vi "WS1050 36 DUT Reliability HD_Cycling_CP CVSweep_Ver1.0.vi"() -> ()   [LabVIEW 2012]
uses:
  WS_VCAP Driver 029/Source/WSVCAP Shell/Type Defs/WSVCAP SHL I2C DUT Mask Mode Enum.ctl
  <vilib>/Utility/file.llb/Read From Spreadsheet File (DBL).vi
panel:
  out "VISA out":refnum<visa-resource-name>="GPIB0::3::INSTR"
  out "error out 2":errorcluster={"status"=TRUE, "code"=-63192, "source"="niLvFpga_Open_PXI-7813R.vi"}
  in  "Reg1_Bit Cntrl":string[](array[string])=["01", "02", "04", "08", "10", "20", "40", "80", "03", "06", "0C", "D8", "33", "66", "CC", "07", "0E", "1C", "38", "70", "E0", "0F", "1E", "3C", "78", "F0", "1F", "3E", "7C", "F8", "3F", "7E", "FC", "7F", "FE", "FD", "FB", "F7", "EF", "DF", "BF", "7F", "FC", "F9", "F3", "E7", "CF", "9F", "3F", "F8", "F1", "E3", "C7", "8F", "1F", "F0", "E1", "C3", "87", "0F", "E0", "C1", "83", "07", "C0", "81", "03", "AA", "55", "00"]
  out "date string":string="5/19/2014"
  out "PS1 Out":refnum<visa-resource-name>
  out "Ke2000 Out":refnum<visa-resource-name>="GPIB0::9::INSTR"
  in  "VPI_Cmd":string[](array[string])=["00", "3B", "00"]
  in  "VPI Name":string[](array[string])=["All_Drivers OFF", "All Drivers ON", "All Drivers OFF2"]
  in  "Tab Control":T1(tab)
  in  "CP with DVA ON":i32(ring) items=["CP HDC 35V", "CP HDC 40.25V", "CP HDC 27.5V", "CP HDC 30.5V", "CP HDC 44V", "CP HDC 50V", "CP HDC 55V", "CP HDC 42.5V", "CP HDC 32V"]
  in  "No of Cmd":i64=2
  in  "Board#":string="BRD5"
  in  "Serial Number":string[][](table)=[["DUT", "SN"], ["DUT1", "1"], ["DUT2", "2"], ["DUT3", "3"], ["DUT4", "4"], ["DUT5", "5"], ["DUT6", "6"], ["DUT7", "7"], ["DUT8", "8"], ["DUT9", "9"], ["DUT10", "10"], ["DUT11", "11"], ["DUT12", "12"], ["DUT13", "13"], ["DUT14", "14"], ["DUT15", "15"], ["DUT16", "16"], ["DUT17", "17"], ["DUT18", "18"], ["DUT19", "19"], ["DUT20", "20"], ["DUT21", "21"], ["DUT22", "22"], ["DUT23", "23"], ["DUT24", "24"], ["DUT25", "25"], ["DUT26", "26"], ["DUT27", "27"], ["DUT28", "28"], ["DUT29", "29"], ["DUT30", "30"], ["DUT31", "31"], ["DUT32", "32"], ["DUT33", "33"], ["DUT34", "34"], ["DUT35", "35"], ["DUT36", "36"]]
  in  "SPI Clock Rate (Hz)":dbl=5000000.0 caption="Cycle Speed" format="%.1p Hz"
  in  "Wafer#":string="T7-EB"
  in  "File Name":string="CYC_WS1050_T7_EB_65C_40V_25DC_BRD5_150911_1"
  in  "TMN DC\\CAP Data Log File Path":path=path "C:/WS1050 36 DUT Data"
  in  "Test Program":string="WS1050 36 DUT HD_Cycling_CP CV Sweep Ver1.0"
  out "Current Date":string="8/28/2014"
  out "Current Time":string="0950"
  in  "Start Date":string="10/21/2014"
  in  "Start Time":string="1542"
  in  "Comment":string="CYC65C40V"
  in  "OK Button":bool
  in  "Calibration":bool
  in  "Verify CP":bool
  in  "CP Setting":i32(ring) items=["CP OFF", "CP ON", "CP 35V", "CP 40V", "DVA ON", "DVA OFF", "REG1 ON", "REG1 OFF", "REG2 ON", "REG2 OFF", "REG3 ON", "REG3 OFF"]
  in  "Set VDD":dbl=3.7 format="%.3g"
  in  "Command":string[](array[string])=["0702013B3B3B", "070201000000", "0702013B0000"]
  in  "Clock Rate (Hz)":dbl=1000000.0 caption="Meas Speed" format="%.1p Hz"
  out "AR  Measurent(Hz)":dbl
  in  "PS1 Source":refnum<visa-resource-name>="GPIB0::5::INSTR"
  in  "Ke2000":refnum<visa-resource-name>="GPIB0::9::INSTR"
  in  "CP to HD/Cycle":i32(ring)=1 items=["CP HDC 35V", "CP HDC 40.25V", "CP HDC 27.5V", "CP HDC 30.5V", "CP HDC 44V", "CP HDC 50V", "CP HDC 55V", "CP HDC 42.5V", "CP HDC 32V"]
  out "Simulate FPGA":bool
  out "Online":bool
  out "AR Cycling(Hz)":dbl=5000000.0
  in  "Ke2400":refnum<visa-resource-name>="GPIB0::3::INSTR"
  in  "Initialize AD7747":bool
  in  "DUT Mask Mode":T2=enum."All"
  in  "RFFE Slave Address":u8=7 caption="Slave Address" format="0x%02x"
  out "Activity Log":string="05/19/2014 -- 12:24:35.853::WSVCAP::APP::Application Started\n05/19/2014 -- 12:24:37.606::WSVCAP::WSVCAP SHL::WR I2C-REG:0x0A;MASK:0xFFFFFFFFFFFF;C1 DATA:22:22:22:22:22:22:22:22:22:22:22:22:22:22:22:22;C2 DATA:22:22:22:22:22:22:22:22:22:22:22:22:22:22:22:22;C3 DATA:22:22:22:22:22:22:22:22:22:22:22:22:22:22:22:22\r\n05/19/2014 -- 12:24:37.773::WSVCAP::WSVCAP SHL::WR I2C-ST:0,0,4,1\r\n05/19/2014 -- 12:24:37.903::WSVCAP::WSVCAP SHL::RD I2C-BYTES:4;ADD:0x00;MASK:0xFFFFFFFFFFFF\r\n05/19/2014 -- 12:24:38.045::WSVCAP::WSVCAP SHL::RD I2C:C1 DATA:2:2:2:2:2:2:2:2:2:2:2:2:2:2:2:2|A7:A9:AA:82:82:7F:82:81:82:81:83:82:81:82:82:81|46:36:BB:88:44:A3:E9:2B:32:20:ED:25:BB:3D:68:B|2C:6A:EB:A7:22:56:FE:CC:36:82:D7:B0:3B:48:F9:CC;C2 DATA:2:2:2:2:2:2:2:2:2:2:2:2:2:2:2:2|94:94:94:80:80:80:80:80:81:7E:7E:81:80:7E:80:80|47:33:15:82:62:B:E8:1C:D7:C3:7D:41:7C:B7:4C:2A|C4:B4:AE:8:1E:D1:4E:37:11:C0:6F:63:42:9D:63:B5;C3 DATA:2:2:2:2:2:2:2:2:2:2:2:2:2:2:2:2|95:95:95:81:81:7E:81:80:84:7D:80:83:81:7E:7F:80|AB:C4:14:B5:7B:52:DF:C9:79:5D:5F:30:99:31:1E:F4|6E:5C:F7:A8:C3:EB:7B:EF:33:92:89:77:4D:67:75:DD;STATUS:0:0:4:0\r\n05/19/2014 -- 12:24:38.046::WSVCAP::WSVCAP SHL::WR I2C-REG:0x0A;MASK:0xFFFFFFFFFFFF;C1 DATA:22:22:22:22:22:22:22:22:22:22:22:22:22:22:22:22;C2 DATA:22:22:22:22:22:22:22:22:22:22:22:22:22:22:22:22;C3 DATA:22:22:22:22:22:22:22:22:22:22:22:22:22:22:22:22\r\n05/19/2014 -- 12:24:38.089::WSVCAP::WSVCAP SHL::WR I2C-ST:0,0,4,1\r\n05/19/2014 -- 12:24:38.219::WSVCAP::WSVCAP SHL::RD I2C-BYTES:4;ADD:0x00;MASK:0xFFFFFFFFFFFF\r\n05/19/2014 -- 12:24:38.362::WSVCAP::WSVCAP SHL::RD I2C:C1 DATA:2:2:2:2:2:2:2:2:2:2:2:2:2:2:2:2|A7:AB:AA:82:82:82:83:83:82:82:82:82:7F:82:82:81|4B:32:96:83:3E:61:43:17:25:62:AB:4D:A2:40:2E:5|3C:76:2B:B4:EE:E4:A9:1A:AA:A:26:C7:21:2E:87:5B;C2 DATA:2:2:2:2:2:2:2:2:2:2:2:2:2:2:2:2|94:94:94:80:80:80:80:80:80:7F:80:81:80:80:7F:80|4A:32:19:7D:19:6C:79:46:61:7F:4B:B8:A5:30:F3:14|B4:70:A:8C:9C:DC:43:FA:1E:A:C6:21:A:A9:13:F3;C3 DATA:2:2:2:2:2:2:2:2:2:2:2:2:2:2:2:2|95:97:94:81:80:81:82:81:80:7E:81:84:7F:81:80:80|B2:32:D0:A7:9E:4C:AB:D4:EE:D9:F0:82:B7:91:7:FF|C1:91:B6:3D:D8:E:1B:4F:9F:6A:F1:6C:E7:3F:7:BA;STATUS:0:0:4:0\r\n05/19/2014 -- 12:24:38.364::WSVCAP::WSVCAP SHL::WR I2C-REG:0x0A;MASK:0xFFFFFFFFFFFF;C1 DATA:22:22:22:22:22:22:22:22:22:22:22:22:22:22:22:22;C2 DATA:22:22:22:22:22:22:22:22:22:22:22:22:22:22:22:22;C3 DATA:22:22:22:22:22:22:22:22:22:22:22:22:22:22:22:22\r\n05/19/2014 -- 12:24:38.406::WSVCAP::WSVCAP SHL::WR I2C-ST:0,0,4,1\r\n05/19/2014 -- 12:24:38.536::WSVCAP::WSVCAP SHL::RD I2C-BYTES:4;ADD:0x00;MASK:0xFFFFFFFFFFFF\r\n05/19/2014 -- 12:24:38.678::WSVCAP::WSVCAP SHL::RD I2C:C1 DATA:2:2:2:2:2:2:2:2:2:2:2:2:2:2:2:2|A7:A9:AB:82:82:81:82:82:82:82:82:82:82:82:82:81|46:71:4C:87:43:3D:7F:FC:25:4F:8E:54:97:3E:60:8C|AA:F4:1F:B5:CE:43:1F:36:9:87:9C:78:86:5:B6:8E;C2 DATA:2:2:2:2:2:2:2:2:2:2:2:2:2:2:2:2|94:94:94:80:7F:7F:80:80:80:80:80:81:80:80:80:80|49:36:18:7D:6E:C5:E4:3C:81:2E:41:D3:75:71:E3:72|E8:D3:E6:D1:E0:48:AE:D4:54:D:E8:8E:B4:41:68:4;C3 DATA:2:2:2:2:2:2:2:2:2:2:2:2:2:2:2:2|95:95:95:81:7F:7F:81:81:81:81:81:84:81:81:82:81|B3:F5:90:AB:82:69:7B:93:D0:77:E8:D5:E8:8C:84:E8|B9:AC:EE:2B:B6:71:8F:4A:74:31:56:BB:8A:B7:A0:C8;STATUS:0:0:4:0\r\n05/19/2014 -- 12:24:38.681::WSVCAP::WSVCAP SHL::WR I2C-REG:0x0A;MASK:0xFFFFFFFFFFFF;C1 DATA:22:22:22:22:22:22:22:22:22:22:22:22:22:22:22:22;C2 DATA:22:22:22:22:22:22:22:22:22:22:22:22:22:22:22:22;C3 DATA:22:22:22:22:22:22:22:22:22:22:22:22:22:22:22:22\r\n05/19/2014 -- 12:24:38.723::WSVCAP::WSVCAP SHL::WR I2C-ST:0,0,4,1\r\n05/19/2014 -- 12:24:38.854::WSVCAP::WSVCAP SHL::RD I2C-BYTES:4;ADD:0x00;MASK:0xFFFFFFFFFFFF\r\n05/19/2014 -- 12:24:38.996::WSVCAP::WSVCAP SHL::RD I2C:C1 DATA:2:2:2:2:2:2:2:2:2:2:2:2:2:2:2:2|A7:A9:AA:82:82:7F:83:81:82:81:84:82:7F:82:7F:82|43:FB:E:7F:3C:AD:35:35:26:A2:6C:21:4B:3D:8:6|63:9A:E1:F3:95:32:91:42:90:3C:78:1F:5C:D7:5F:D8;C2 DATA:2:2:2:2:2:2:2:2:2:2:2:2:2:2:2:2|94:94:94:80:80:80:80:80:81:80:7E:81:80:7E:7F:80|48:36:18:7F:5E:3D:69:83:DE:AE:A1:9E:31:AE:BB:96|15:A0:44:17:13:FD:CC:C8:6D:B2:EF:A7:C:C7:3B:F;C3 DATA:2:2:2:2:2:2:2:2:2:2:2:2:2:2:2:2|95:96:94:81:81:7E:82:80:84:80:80:84:7F:7E:7D:82|AD:3B:6D:A9:7C:57:9D:F5:7A:96:23:5C:36:2D:ED:5A|CD:46:DB:3B:C7:BD:70:60:33:B8:B:F7:63:A:51:4D;STATUS:0:0:4:0\r\n05/19/2014 -- 12:24:38.998::WSVCAP::WSVCAP SHL::WR I2C-REG:0x0A;MASK:0xFFFFFFFFFFFF;C1 DATA:22:22:22:22:22:22:22:22:22:22:22:22:22:22:22:22;C2 DATA:22:22:22:22:22:22:22:22:22:22:22:22:22:22:22:22;C3 DATA:22:22:22:22:22:22:22:22:22:22:22:22:22:22:22:22\r\n05/19/2014 -- 12:24:39.040::WSVCAP::WSVCAP SHL::WR I2C-ST:0,0,4,1\r\n05/19/2014 -- 12:24:39.170::WSVCAP::WSVCAP SHL::RD I2C-BYTES:4;ADD:0x00;MASK:0xFFFFFFFFFFFF\r\n05/19/2014 -- 12:24:39.311::WSVCAP::WSVCAP SHL::RD I2C:C1 DATA:2:2:2:2:2:2:2:2:2:2:2:2:2:2:2:2|A7:AA:AB:82:82:81:82:81:82:81:82:82:82:82:7F:82|44:F1:90:87:45:44:C8:2C:2C:F1:FC:1B:94:3B:3C:75|4A:49:95:19:99:73:64:3:23:24:F3:A2:5E:7F:C4:B6;C2 DATA:2:2:2:2:2:2:2:2:2:2:2:2:2:2:2:2|94:94:94:80:80:80:80:7F:80:80:7E:80:80:7E:7F:80|4C:36:17:7D:A8:9F:DE:C7:53:6D:8A:F4:41:A5:C6:E0|90:2E:24:C:D9:22:E4:76:3B:40:1D:53:33:B1:3E:4D;C3 DATA:2:2:2:2:2:2:2:2:2:2:2:2:2:2:2:2|95:97:95:81:81:7F:81:80:80:81:7F:82:81:7E:7D:82|AE:2B:A7:AB:CC:CD:A4:38:FD:17:80:F2:92:2D:45:C4|76:E5:D:B9:AD:B5:BA:8D:28:32:9E:42:B7:20:4A:D9;STATUS:0:0:4:0\r\n05/19/2014 -- 12:24:39.313::WSVCAP::WSVCAP SHL::WR I2C-REG:0x0A;MASK:0xFFFFFFFFFFFF;C1 DATA:22:22:22:22:22:22:22:22:22:22:22:22:22:22:22:22;C2 DATA:22:22:22:22:22:22:22:22:22:22:22:22:22:22:22:22;C3 DATA:22:22:22:22:22:22:22:22:22:22:22:22:22:22:22:22\r\n05/19/2014 -- 12:24:39.355::WSVCAP::WSVCAP SHL::WR I2C-ST:0,0,4,1\r\n05/19/2014 -- 12:24:39.486::WSVCAP::WSVCAP SHL::RD I2C-BYTES:4;ADD:0x00;MASK:0xFFFFFFFFFFFF\r\n05/19/2014 -- 12:24:39.628::WSVCAP::WSVCAP SHL::RD I2C:C1 DATA:2:2:2:2:2:2:2:2:2:2:2:2:2:2:2:2|A7:A9:AA:82:82:82:83:82:82:82:82:82:7F:82:7F:82|47:18:E4:87:3E:E7:6:65:25:92:37:38:A8:3E:89:85|7C:A7:7:2B:A3:7A:EC:EF:89:ED:F4:D3:D8:BC:3A:F5;C2 DATA:2:2:2:2:2:2:2:2:2:2:2:2:2:2:2:2|94:94:94:80:7F:80:80:7F:81:80:7E:80:80:80:81:80|49:37:17:80:76:25:6A:F8:DF:55:97:4D:B8:5B:2B:B1|13:E3:9A:3E:1A:2D:4F:B6:DB:E9:61:FA:8B:D6:9:CC;C3 DATA:2:2:2:2:2:2:2:2:2:2:2:2:2:2:2:2|95:95:95:81:7F:80:82:81:84:80:7F:81:80:81:7F:82|AF:93:3B:AF:5B:11:82:E4:7E:C3:2D:72:9:96:D9:A|DB:96:F2:10:5F:64:9A:C6:98:12:27:7D:10:D3:20:D9;STATUS:0:0:4:0\r\n05/19/2014 -- 12:24:40.132::WSVCAP::WSVCAP SHL::CLOSE\r\n"
  in  "C1 Cap DAC":u8=128 caption="B Data In" format="0x%02x"
  in  "C2 Cap DAC":u8=128 caption="B Data In" format="0x%02x"
  in  "C3 Cap DAC":u8=128 caption="B Data In" format="0x%02x"
  out "IDD Brd(uA)":string
  in  "Repeat Meas(s)":u32=900
  in  "Real No. From\nLookup Table":bool
  in  "Control Panel":T3={"Verify Socket"=FALSE, "HD/CYC"=FALSE, "E-CAL"=FALSE, "DVA"=FALSE, "VPI"=TRUE, "VSA"=TRUE, "HS"=FALSE}
  out "Verify Socket":bool
  out "HD/CYC":bool
  out "E-CAL":bool
  out "DVA":bool
  out "VPI":bool
  out "VSA":bool
  out "HS":bool
  in  "Lot#":string="WS1050"
  out "AD7747 Values":string[][](table)
  in  "Freq(Hz)":string="12K"
  in  "Reset P/S":bool
  in  "Test Sequences":i32(ring) items=["C1_C2_C3", "C2_C1_C3", "C3_C2_C1"]
  in  "WS1050/51":bool=TRUE
  in  "% Duty Cycle":string="25"
  in  "Cmd To HD":string="0702013B3B3B"
  in  "Post CMd Delay":dbl[](array[numeric])=[1.7e-05, 5.4e-05, 1.8e-05] min=0.0 max=0.5 format="%#.0p s"
  in  "Cmin/Act":bool=TRUE
  in  "CP to Meas":i32(ring)=1 items=["CP HDC 35V", "CP HDC 40.25V", "CP HDC 27.5V", "CP HDC 30.5V", "CP HDC 44V", "CP HDC 50V", "CP HDC 55V", "CP HDC 42.5V", "CP HDC 32V"]
  in  "CP VPI":i32(ring) items=["CP HDC 35V", "CP HDC 40.25V", "CP HDC 27.5V", "CP HDC 30.5V", "CP HDC 44V", "CP HDC 50V", "CP HDC 55V", "CP HDC 42.5V", "CP HDC 32V"]
  out "CAP_C1":string[][](table)
  out "NOM IDD OFF(uA)":string
  out "CAP_C2":string[][](table)
  out "CAP_C3":string[][](table)
  out "Total Time":u64
  in  "Set HD/Cycle \nto Complete":u64=5000000000
  out "No of HD/Cycle\nCompleted":u64
  out "Cycle Count":u64 min=1 max=4 step=1
  out "Loop \ncompleted":i32=1
  out "Previous Time":string="12:20:26 PM"
  out "STATUS":string="Idle...."
  out "Total Delta C2(pF)":string[](array[string])
  out "Total Delta C1(pF)":string[](array[string])
  out "Total Delta C3(pF)":string[](array[string])
  out "RB Reg for HD":string[](array[string])
  out "RB Reg for HD/Cycle":string[](array[string])
  out "VPI C2":string[][](table)
  out "VPI C3":string[][](table)
  out "NOM IDD ON (uA)":string
  out "IDD_HD/CYC (uA)":string="164.601255E+0"
  in  "stop During HD/Cycles":bool
  in  "stop":bool
  out "IDD Stdby(uA)":string="2.606990E+0"
  out "VPI C1":string[][](table)
  out "VSA_V1":string[][](table)
  out "VSA_V2":string[][](table)
  out "VSA_V3":string[][](table)
  in  "VSA Voltage(V)":dbl[](array[numeric])=[-10.0, 0.0, 10.0]
  in  "DC_Temp":i32=65
  in  "HD/CYC Temp":i32=65
  in  "Time All ON (s)":u32=120
  in  "Time All OFF (s)":u32=120
  in  "HD_DC (Min)":u64=259200
  out "LPs Count":i32
  in  "X Repeat":i32=100
  out "No LPs to RP":i32
  out "Run Loops":i32=1
  out "TTCompleted":u64=2000
  in  "TTF Completed":u64=5000000000
  out "% Delta C_T0":string[][](array[string])
  out "% Delta C":string[][](array[string])
  out "EFuse RB T0":string[](array[string])
  out "Current EFuse Read back":string[](array[string])
  out "EFuse Readback Status":bool[](array[boolean])
  in  "DeltaC Target Setting(pF)":dbl=7.375
  out "error out":errorcluster
  in  "error in (no error)":errorcluster
  in  "HD RP":dbl=60.0
  in  "Cycle RP":dbl=10000.0
  out "Min Plot_1":dbl[][](graph) caption="(Y) Multi Plot 2"
  out "Min Plot_2":dbl[][](graph) caption="(Y) Multi Plot 2"
  out "Min Plot_3":dbl[][](graph) caption="(Y) Multi Plot 2"
  in  "Debug":bool
  in  "No of Rows\nFrom Spread Sheet":i32
  in  "Plot Delta Cmin":bool=TRUE
  in  "Plot":T4(ring)
  in  "Bank C1":i32(ring) items=["C1", "C2", "C3", "D_C1", "D_C2", "D_C3"]
  in  "Bank C2":i32(ring)=1 items=["C1", "C2", "C3", "D_C1", "D_C2", "D_C3"]
  in  "Bank C3":i32(ring)=2 items=["C1", "C2", "C3", "D_C1", "D_C2", "D_C3"]
  in  "Manual Setting\nFor RP CP CV":i64[](array[numeric])=[0, 100000, 5000000]
  in  "CP CV \nSweep":bool=TRUE
  out "CP CV Sweep C1":dbl[][](graph) caption="(Y) Multi Plot 2"
  out "CP CV Sweep C2":dbl[][](graph) caption="(Y) Multi Plot 2"
  out "CP CV Sweep C3":dbl[][](graph) caption="(Y) Multi Plot 2"
  out "LP CP Voltage":string
  in  "Auto\nMan":bool
  in  "Start":i64
  in  "Stop":i64
  in  "Step":i64
  out "RP for CP CV":i64[](array[numeric])
  out "CP to Run":dbl[](array[numeric])
  # "Company:  WiSpry Inc\n20 Fairbanks Ste 198 Irvine CA 92618\n\nAuthor:  Andy V Tran\nCreated:  09/14/2015\nLabVIEW 2012 Pro\nTest Program:  WS1050 36 DUT Reliability HD_Cycling CP CV Sweep ver1.0\nFPGA: WS_VCAP Driver 029"
  # "Note for HD Duty Cycle:\n1.  Set time to start HD_DC (Min), default is 259200 (6 months) \n2.  Set Time for Duty Cycle ON/OFF, default setting is 2 minutes\n3.  No of Loops to RP = 3600s/(Time ALL ON(s) + Time ALL + OFF(s))\n4.  Set X Repeat = no of runs, default is 100 runs\n5.  Set TTF Completed to stop the test.\n\nVer 1.0:\n1.  Original version, set CP voltage measure all drivers"
  # "Minutes"
  # "X1000"
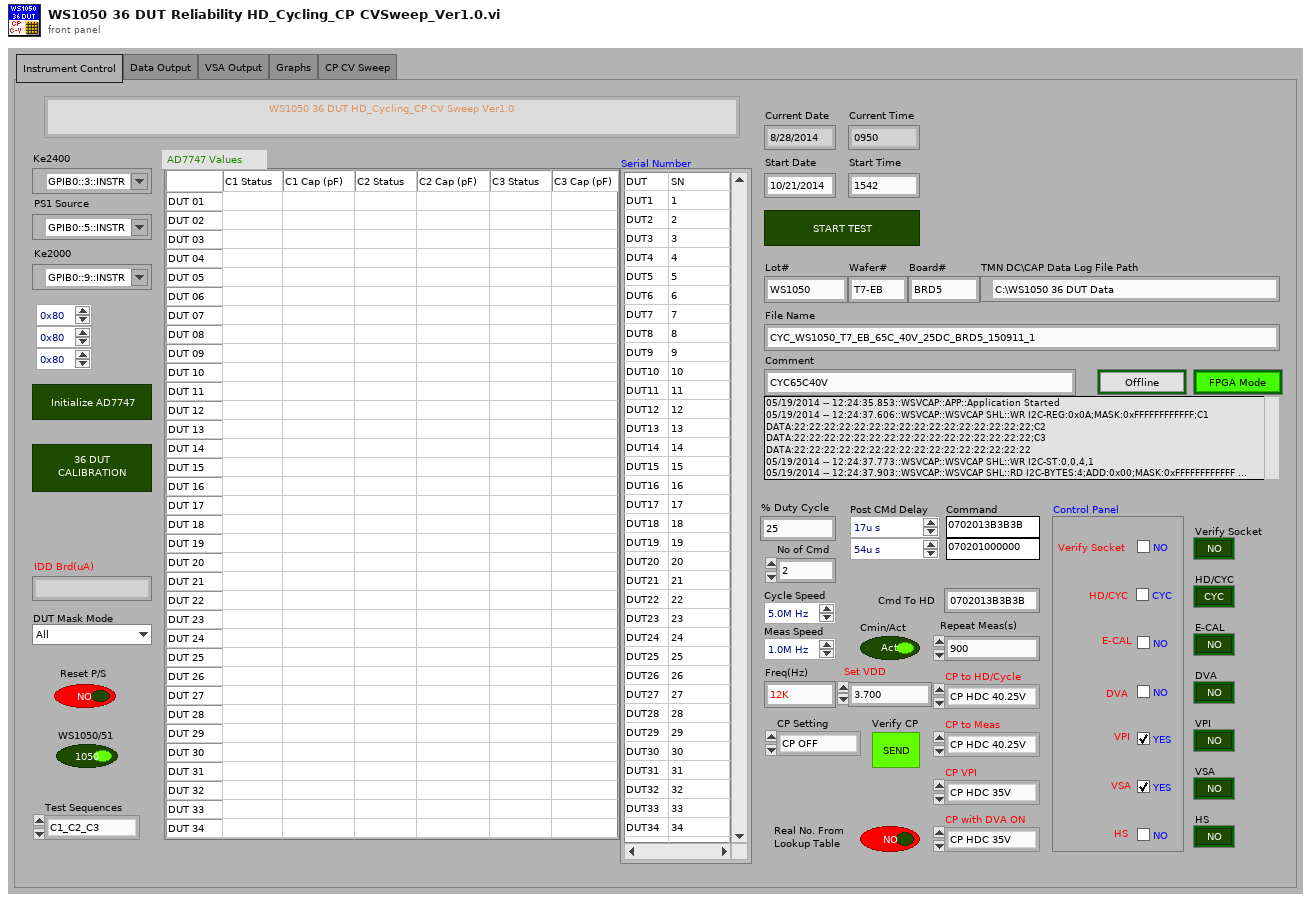
[diagram p1: front panel]
types:
  T1 = enum32{"Instrument Control", "Data Output", "VSA Output", "Graphs", "CP CV Sweep"}
  T2 = typedef "WSVCAP SHL I2C DUT Mask Mode Enum.ctl" = enum16{"Custom", "C1", "C2", "C3", "All"}
  T3 = cluster{"Verify Socket":bool, "HD/CYC":bool, "E-CAL":bool, "DVA":bool, "VPI":bool, "VSA":bool, "HS":bool}
  T4 = enum16{"ALL DUTs", "DUT 01", "DUT 02", "DUT 03", "DUT 04", "DUT 05", "DUT 06", "DUT 07", "DUT 08", "DUT 09", "DUT 10", "DUT 11", "DUT 12", "DUT 13", "DUT 14", "DUT 15", "DUT 16", "DUT 17", "DUT 18", "DUT 19", "DUT 20", "DUT 21", "DUT 22", "DUT 23", "DUT 24", "DUT 25", "DUT 26", "DUT 27", "DUT 28", "DUT 29", "DUT 30", "DUT 31", "DUT 32", "DUT 33", "DUT 34", "DUT 35", "DUT 36"}
  T5 = typedef "WSVCAP SHL Core System Cluster.ctl" = cluster{"Settings":T6, "FPGA Resource":tag, "Online":bool, "I2C Wait Ticks":u32, "SPI Wait Ticks":u32, "RFFE Wait Ticks":u32}
  T6 = typedef "WSVCAP SHL I2C Settings Cluster.ctl" = cluster{"FPGA Resource Name":string, "I2C Slave Address":u8, "I2C Clock Rate (Hz)":dbl, "SPI Clock Rate (Hz)":dbl, "RFFE Slave Address":u8, "RFFE Clock Rate (Hz)":dbl, "Simulate FPGA":bool, "C1 Cap DAC Default":u8, "C2 Cap DAC Default":u8, "C3 Cap DAC Default":u8}
  T7 = enum16{"Idle...", "Voltage 1", "Voltage 2", "Voltage 3"}[]
  T8 = cluster{"Test Program ":string, "Comment":string, "Data Out":string, "Data Out":string, "Data Out":string, string, "Data Out":string, "Data Out":string, "Data Out":string, "Freq(Hz)":string, "Board#":string}
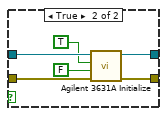
[diagram p2: hidden frame]
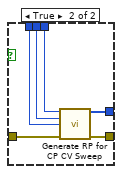
[diagram p8: hidden frame]
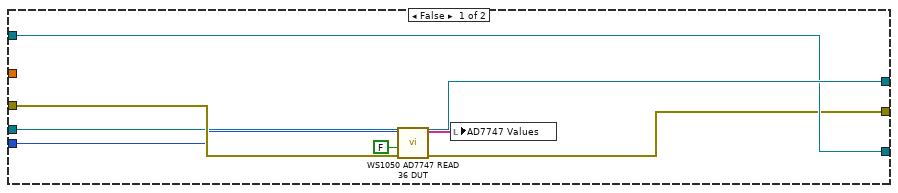
[diagram p11: hidden frame]
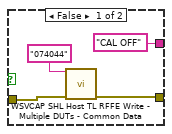
[diagram p12: hidden frame]
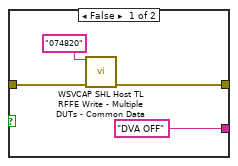
[diagram p13: hidden frame]
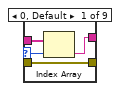
[diagram p14: hidden frame]
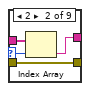
[diagram p15: hidden frame]
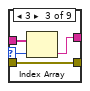
[diagram p16: hidden frame]
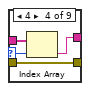
[diagram p17: hidden frame]
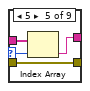
[diagram p18: hidden frame]
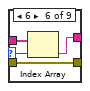
[diagram p19: hidden frame]
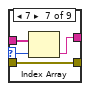
[diagram p20: hidden frame]
diagram:
  w26 = TRUE
  w30 = u16 0 items=["Off", "Moving Filter", "Repeating Filter"] ("Digital Filter (0: Off)")
  w31 = u16 7 items=["3.5 Digits"=4, "4.5 Digits"=5, "5.5 Digits"=6, "6.5 Digits"=7] ("Resolution (7: 6.5 digits)")
  n1 = case shown="True" w26 {
    tunnel: "error in (no error)" -> [w38 w39]
    tunnel: [w38 w46] -> w15
    frame False {
    }
    frame True {
      n2 = call "WSVCAP SHL Host TL Initialize.vi"("error in"=w39) -> ("error out"=w40:errorcluster)  [unwired: 13 in, 1 out]
      n3 = control-ref of="Activity Log"() -> (w42:refnum<vi>)
      n4 = call "ACT LG Activity Log Core.vi"("Display Ref"=w42, "Source"="WSVCAP", "Error In (no error)"=w40) -> ("Error Out"=w41:errorcluster)  [unwired: 11 in, 1 out]
      n5 = call "WSVCAP SHL Host TL Status Manager.vi"("error in"=w41) -> ("System Out"=w47:T5, "error out"=w46:errorcluster)  [unwired: 13 in]
      n6 = Unbundle By Name(w47) -> ("Online"=→"Online":bool, "Settings.Simulate FPGA"=→"Simulate FPGA":bool)
    }
  }
  n7 = case shown="True" TRUE {
    tunnel: [_ w50] -> w37
    tunnel: [_ w48] -> w1
    frame False {
    }
    frame True {
      n8 = flat-sequence {
        tunnel: [w51] -> w49
        tunnel: [w55] -> w50
        tunnel: w49 -> [w55]
        tunnel: [w53] -> w48
        frame #0 {
          n9 = call-poly <vilib>:"Read From Spreadsheet File.vi"("number of rows (all:-1)"=-1) -> ("all rows"=w51:dbl[][])  [unwired: 6 in, 4 out]
        }
        frame #1 {
          n10 = call-poly <vilib>:"Read From Spreadsheet File.vi"("number of rows (all:-1)"=-1) -> ("all rows"=w53:dbl[][])  [unwired: 6 in, 4 out]
        }
      }
    }
  }
  n11 = case shown="True" TRUE {
    tunnel: w15 -> [w56 w61]
    tunnel: [w57 w60] -> w23
    tunnel: [w56 w59] -> w19
    tunnel: "Ke2400" -> [w57 w58]
    frame False {
    }
    frame True {
      n12 = VISA Write(VISA resource name=w58, write buffer="SOUR:FUNC VOLT;VOLT:MODE FIX;RANG 100;LEV 0.0;:SENS:FUNC \"CURR\";CURR:PROT 60E-3;RANG 100E-3;:OUTP ON", error in (no error)=w61) -> (VISA resource name out=w60:refnum<visa-resource-name>, error out=w59:errorcluster)  [unwired: 1 out]
    }
  }
  n13 = case shown="False" "Reset P/S" {
    tunnel: "PS1 Source" -> [w63 w70]
    tunnel: [w63 w68] -> w35
    tunnel: w15 -> [w64 w66]
    tunnel: [w64 w65] -> w14
    frame False {
    }
    frame True {
      n14 = call "Agilent 3631A Initialize.vi"("error in (no error)"=w66, "Default"=FALSE ("Reset? (T: Yes)"), "Reset"=TRUE ("ID Query? (T: Yes)"), "VISA resource name"=w70) -> ("error out"=w65:errorcluster, "VISA resource name out"=w68:refnum<visa-resource-name>)  [unwired: 6 in]
    }
  }
  n15 = call "Ke2000 Initialize.vi"("error in (no error)"=w15, "VISA resource name"="Ke2000") -> ("error out"=w32:errorcluster, "VISA resource name out"=w33:refnum<visa-resource-name>)  [unwired: 8 in]
  n16 = call "Ke2000 Configure DC Current.vi"("Resolution (7: 6.5 digits)"=w31, "Digital Filter (0: Off)"=w30, "Auto Range? (T: Auto)"=FALSE, "error in"=w32, "Custom Range (0 A)"=1.0, "VISA resource name"=w33) -> ("error out"=w16:errorcluster, "VISA resource name out"=w28:refnum<visa-resource-name>)  [unwired: 4 in]
  n17 = Merge Errors(w19, w16, w14) -> (w24:errorcluster)
  n18 = while {
    tunnel: w24 -> [w79]
    tunnel: [w75] -> w5
    tunnel: w37 -> [w102]
    tunnel: w35 -> [w90]
    tunnel: w28 -> [w91]
    tunnel: [w100] -> w11
    tunnel: [w99] -> w6
    tunnel: w23 -> [w97]
    tunnel: [w96] -> w21
    tunnel: [FALSE ("stop")] -> w17
    tunnel: w1 -> [w72]
    i -> [w98]
    stop <- w103 stop-if-true
    n19 = case shown="0" w98 {
      tunnel: w79 -> [w113 w115]
      tunnel: [w112 w115] -> w93
      tunnel: "RFFE Slave Address" -> [w110 _]
      frame 0 {
        w106 = dbl[][] []
        w105 = "" ("uA")
        w107 = string[][] []
        w108 = string[] [] ("EFuse Read back")
        w114 = u64 0 ("No of HD/Cycle\nCompleted")
        n20 = local write "RB Reg for HD/Cycle"(w108) -> ()
        n21 = local write "Current EFuse Read back"(w108) -> ()
        n22 = local write "EFuse RB T0"(w108) -> ()
        n23 = local write "Total Delta C1(pF)"(w108) -> ()
        n24 = local write "Total Delta C2(pF)"(w108) -> ()
        n25 = local write "Total Delta C3(pF)"(w108) -> ()
        n26 = local write "No of HD/Cycle\nCompleted"(w114) -> ()
        n27 = local write "Cycle Count"(w114) -> ()
        n28 = local write "CAP_C2"(w107) -> ()
        n29 = local write "CAP_C1"(w107) -> ()
        n30 = local write "VPI C2"(w107) -> ()
        n31 = local write "VSA_V3"(w107) -> ()
        n32 = local write "VSA_V1"(w107) -> ()
        n33 = local write "NOM IDD OFF(uA)"(w105) -> ()
        n34 = local write "NOM IDD ON (uA)"(w105) -> ()
        n35 = local write "IDD Brd(uA)"(w105) -> ()
        n36 = local write "CAP_C3"(w107) -> ()
        n37 = local write "VSA_V2"(w107) -> ()
        n38 = local write "VPI C1"(w107) -> ()
        n39 = local write "VPI C3"(w107) -> ()
        n40 = local write "% Delta C"(w107) -> ()
        n41 = local write "% Delta C_T0"(w107) -> ()
        n42 = call "WSVCAP SHL Host TL RFFE Configure.vi"("RFFE Slave Address"=w110, "Clock Rate (Hz)"="Clock Rate (Hz)", "error in"=w113) -> ("Actual Rate (Hz)"=→"AR  Measurent(Hz)":dbl, "error out"=w112:errorcluster)  [unwired: 11 in]
        n43 = local write "Min Plot_3"(w106) -> ()
        n44 = local write "Min Plot_1"(w106) -> ()
        n45 = local write "Min Plot_2"(w106) -> ()
      }
      frame 1, Default {
      }
    }
    n46 = while {
      tunnel: ["stop"] -> w95
      tunnel: w93 -> [w152]
      tunnel: [w121] -> w87
      tunnel: w90 -> [w151]
      tunnel: w91 -> [w146]
      tunnel: [w147] -> w89
      tunnel: [w145] -> w88
      tunnel: [w143] -> w86
      tunnel: [w142] -> w85
      tunnel: [w141] -> w84
      tunnel: [w140] -> w83
      tunnel: [w139] -> w82
      tunnel: [w138] -> w81
      tunnel: [w137] -> w80
      tunnel: ["Command"] -> w78
      tunnel: ["Post CMd Delay"] -> w77
      tunnel: "Set VDD" -> [w127]
      tunnel: [w116] -> w71
      stop <- w159 stop-if-true
      # "Set Date & Time to Start Test"
      n47 = case shown="True" "Initialize AD7747" {
        tunnel: w152 -> [w176 w182]
        tunnel: [w176 w178] -> w136
        tunnel: w151 -> [w175 w180]
        tunnel: [w175 w179] -> w150
        tunnel: w127 -> [_ w177]
        frame False {
        }
        frame True {
          w183 = T7 [enum."Voltage 2", enum."Voltage 3", enum."Voltage 1"] items=["Idle...", "Voltage 1", "Voltage 2", "Voltage 3"]
          n48 = for {
            tunnel: w180 -> [w193]
            tunnel: w183 -> [w191] mode=indexing
            tunnel: [w190] -> w179
            shift-right: [w187] -> w181
            shift-left: w182 -> [w194]
            tunnel: w177 -> [w184]
            n49 = call "E3631A_Voltage Controller updated.vi"("VISA resource name"=w193, "I_VDD(A)"=0.5, "Channel Controller"=w191, "Voltage 1"=w184, "Voltage 2"=3.3, "error in (no error)"=w194, "I_3.3V (A)"=0.5) -> ("VISA resource name out"=w190:refnum<visa-resource-name>, "error out"=w186:errorcluster)  [unwired: 7 in]
            n50 = call "Delay.vi"("milliseconds to wait"=u32 100, "error in (no error)"=w186) -> ("error out"=w187:errorcluster)  [unwired: 9 in]
          }
          n51 = call "WS1050_AD7747_Init 36DUT.vi"("error in"=w181) -> ("error out"=w178:errorcluster)  [unwired: 10 in]
        }
      }
      n52 = call "Time_stamp.vi"() -> ("date/time string"=w164:string, "date string"=w166:string)  [unwired: 2 in]
      "Current Date" <- w166
      "Current Time" <- w164
      n53 = Equal?(x=w166, y="Start Date") -> (x = y?=w162:bool)
      n54 = Equal?(x=w164, y="Start Time") -> (x = y?=w161:bool)
      n55 = And(x=w162, y=w161) -> (x .and. y?=w158:bool)
      n56 = Compound Arithmetic op=OR(w158, "OK Button", "stop") -> (w159:bool)
      n57 = case shown="True" "Calibration" {
        tunnel: w136 -> [w225 w243]
        tunnel: [w219 w240] -> w134
        tunnel: w150 -> [w224 w239]
        tunnel: "DUT Mask Mode" -> [w223 w235]
        tunnel: [w224 w234] -> w148
        tunnel: w146 -> [w222 w233]
        tunnel: [w222 w230] -> w145
        tunnel: w127 -> [_ w229]
        tunnel: "C1 Cap DAC" -> [_ w228]
        tunnel: "C2 Cap DAC" -> [_ w227]
        tunnel: "C3 Cap DAC" -> [_ w226]
        frame False {
          n58 = call "WS1050 AD7747 READ 36 DUT.vi"("error in"=w225, "Log (T)"=FALSE, "DUT Mask Mode (All)"=w223) -> ("error out"=w219:errorcluster, "AD7747 Values"=w220:string[][])  [unwired: 7 in]
          n59 = local write "AD7747 Values"(w220) -> ()
        }
        frame True {
          n60 = flat-sequence {
            tunnel: w243 -> [w253]
            tunnel: [w248] -> w242
            tunnel: w239 -> [w252]
            tunnel: [w251] -> w238
            tunnel: w235 -> [w250]
            tunnel: [w250] -> w236
            tunnel: w233 -> [w246]
            tunnel: [w245] -> w232
            tunnel: w229 -> [w244]
            tunnel: w242 -> [w279]
            tunnel: [w278] -> w241
            tunnel: w238 -> [w277]
            tunnel: [w277] -> w237
            tunnel: w236 -> [w276]
            tunnel: w228 -> [w272]
            tunnel: w227 -> [w271]
            tunnel: w226 -> [w270]
            tunnel: w232 -> [w269]
            tunnel: [w269] -> w231
            tunnel: w241 -> [w282]
            tunnel: [w285] -> w240
            tunnel: w237 -> [w284]
            tunnel: [w281] -> w234
            tunnel: w231 -> [w280]
            tunnel: [w280] -> w230
            frame #0 {
              w254 = T7 [enum."Voltage 2", enum."Voltage 3", enum."Voltage 1"] items=["Idle...", "Voltage 1", "Voltage 2", "Voltage 3"]
              n61 = for {
                tunnel: w252 -> [w265]
                tunnel: w254 -> [w263] mode=indexing
                tunnel: [w262] -> w251
                shift-right: [w260] -> w247
                shift-left: w253 -> [w266]
                tunnel: w244 -> [w256]
                n62 = call "E3631A_Voltage Controller updated.vi"("VISA resource name"=w265, "I_VDD(A)"=0.5, "Channel Controller"=w263, "Voltage 1"=w256, "Voltage 2"=3.3, "error in (no error)"=w266, "I_3.3V (A)"=0.5) -> ("VISA resource name out"=w262:refnum<visa-resource-name>, "error out"=w259:errorcluster)  [unwired: 7 in]
                n63 = call "Delay.vi"("milliseconds to wait"=u32 100, "error in (no error)"=w259) -> ("error out"=w260:errorcluster)  [unwired: 9 in]
              }
              n64 = call "Ke2000 Single Reading.vi"("error in (no error)"=w247, "VISA resource name"=w246) -> ("error out"=w248:errorcluster, "VISA resource name out"=w245:refnum<visa-resource-name>, "uA"=→"IDD Brd(uA)":string)  [unwired: 5 in, 2 out]
              n65 = One Button Dialog(message="Please verify all sockets should be empty...") -> ()  [unwired: 1 in, 1 out]
            }
            frame #1 {
              n66 = call "WS1050 CAPDAC Setting.vi"("DUT Mask Mode (All)"=w276, "error in"=w279, "C3 Cap DAC"=w270, "C2 Cap DAC"=w271, "C1 Cap DAC"=w272) -> ("error out"=w274:errorcluster)  [unwired: 6 in]
              n67 = call "WS1050 OFFSET CAL updated.vi"("error in"=w274, "OFFSET CAL"=TRUE ("Read?")) -> ("error out"=w273:errorcluster)  [unwired: 9 in]
              n68 = call "WS1050 AD7747 READ 36 DUT.vi"("error in"=w273, "Log (T)"=FALSE, "DUT Mask Mode (All)"=w276) -> ("error out"=w278:errorcluster, "AD7747 Values"=→"AD7747 Values":string[][])  [unwired: 7 in]
            }
            frame #2 {
              w283 = T7 [enum."Voltage 2", enum."Voltage 3", enum."Voltage 1"] items=["Idle...", "Voltage 1", "Voltage 2", "Voltage 3"]
              n69 = for {
                tunnel: w284 -> [w297]
                tunnel: w283 -> [w294] mode=indexing
                tunnel: [w293] -> w281
                shift-right: [w289] -> w285
                shift-left: w282 -> [w295]
                n70 = call "E3631A_Voltage Controller updated.vi"("VISA resource name"=w297, "I_VDD(A)"=0.5, "Channel Controller"=w294, "Voltage 1"=0.0, "Voltage 2"=3.3, "error in (no error)"=w295, "I_3.3V (A)"=0.5) -> ("VISA resource name out"=w293:refnum<visa-resource-name>, "error out"=w288:errorcluster)  [unwired: 7 in]
                n71 = call "Delay.vi"("milliseconds to wait"=u32 100, "error in (no error)"=w288) -> ("error out"=w289:errorcluster)  [unwired: 9 in]
              }
              n72 = One Button Dialog(message="Calibration Completed....") -> ()  [unwired: 1 in, 1 out]
            }
          }
        }
      }
      n73 = local write "stop During HD/Cycles"(FALSE ("stop During HD/Cycles")) -> ()
      n74 = call "Control Panel.vi"("error in (no error)"=w136, "Control Panel"="Control Panel") -> ("error out"=w133:errorcluster, "VPI"=w139:bool, "DVA"=w140:bool, "E-CAL"=w141:bool, "VSA"=w138:bool, "HD/CYC"=w142:bool, "HS"=w137:bool, "Verify Socket"=w143:bool)  [unwired: 2 in]
      "Verify Socket" <- w143
      "E-CAL" <- w141
      "VPI" <- w139
      "VSA" <- w138
      "HS" <- w137
      "HD/CYC" <- w142
      "DVA" <- w140
      n75 = Merge Errors(w133, w134) -> (w135:errorcluster)
      n76 = case shown="True" "Verify CP" {
        tunnel: [w195 w200] -> w122
        tunnel: w148 -> [w196 w203]
        tunnel: [w196 w201] -> w147
        tunnel: w135 -> [w195 w199]
        tunnel: w127 -> [_ w197]
        frame False {
        }
        frame True {
          w204 = T7 [enum."Voltage 2", enum."Voltage 3", enum."Voltage 1"] items=["Idle...", "Voltage 1", "Voltage 2", "Voltage 3"]
          # "Verify CP"
          n77 = for {
            tunnel: w203 -> [w217]
            tunnel: w204 -> [w215] mode=indexing
            shift-right: [w213] -> w202
            shift-left: w199 -> [w218]
            tunnel: [w211] -> w201
            tunnel: w197 -> [w208]
            n78 = call "E3631A_Voltage Controller updated.vi"("VISA resource name"=w217, "I_VDD(A)"=0.5, "Channel Controller"=w215, "Voltage 1"=w208, "Voltage 2"=3.3, "error in (no error)"=w218, "I_3.3V (A)"=0.5) -> ("VISA resource name out"=w211:refnum<visa-resource-name>, "error out"=w214:errorcluster)  [unwired: 7 in]
            n79 = call "Delay.vi"("milliseconds to wait"=u32 100, "error in (no error)"=w214) -> ("error out"=w213:errorcluster)  [unwired: 9 in]
          }
          n80 = Index Array(array=string[] ["074000", "074040", "07476F", "074776", "074800", "074820", "07413B", "074100", "07423B", "074200", "07433B", "074300"], index="CP Setting") -> (element=w205:string)
          n81 = call "WSVCAP SHL Host TL RFFE Write - Multiple DUTs - Common Data.vi"("Data Out"=w205, "error in"=w202, "Log (T)"=FALSE) -> ("error out"=w200:errorcluster)  [unwired: 12 in]
        }
      }
      n82 = Array Subset(array="Post CMd Delay", length="No of Cmd") -> (w131:dbl[])  [unwired: 1 in]
      n83 = Array Subset(array="Command", length="No of Cmd") -> (w132:string[])  [unwired: 1 in]
      n84 = property on="Post CMd Delay" class="Arr (strict)"("Number of Rows"="No of Cmd") -> ()  [unwired: 2 in, 2 out]
      n85 = local write "Command"(w132) -> ()
      n86 = local write "Post CMd Delay"(w131) -> ()
      n87 = property on="Command" class="Arr (strict)"("Number of Rows"="No of Cmd") -> ()  [unwired: 2 in, 2 out]
      n88 = case shown="False" "Auto\nMan" {
        tunnel: w122 -> [w168 w174]
        tunnel: [w168 w173] -> w121
        tunnel: "Start" -> [_ w172]
        tunnel: "Stop" -> [_ w170]
        tunnel: "Step" -> [_ w171]
        tunnel: ["Manual Setting\nFor RP CP CV" w169] -> w116
        frame False {
        }
        frame True {
          n89 = call "Generate RP for CP CV Sweep.vi"("Start"=w172, "Step"=w171, "Stop"=w170, "error in (no error)"=w174) -> ("RP for CP CV"=w169:i64[], "error out"=w173:errorcluster)  [unwired: 10 in]
        }
      }
      "RP for CP CV" <- w116
      n90 = Wait Until Next ms Multiple(millisecond multiple=u32 100) -> ()  [unwired: 1 out]
    }
    n91 = case shown="False" w95 {
      tunnel: w87 -> [w365 w2183]
      tunnel: [w350 w2183] -> w75
      tunnel: w102 -> [w366 _]
      tunnel: w89 -> [w364 w2181]
      tunnel: w88 -> [w356 w2182]
      tunnel: [w362 w2182] -> w100
      tunnel: [w360 w2181] -> w99
      tunnel: w97 -> [w353 w2180]
      tunnel: [w349 w2180] -> w96
      tunnel: "RFFE Slave Address" -> [w344 _]
      tunnel: [FALSE ("stop During HD/Cycles") w2179] -> _
      tunnel: w86 -> [w322 _]
      tunnel: w85 -> [w321 _]
      tunnel: w84 -> [w320 _]
      tunnel: w83 -> [w319 _]
      tunnel: w82 -> [w318 _]
      tunnel: w81 -> [w317 _]
      tunnel: w80 -> [w316 _]
      tunnel: w78 -> [w310 _]
      tunnel: w77 -> [w309 _]
      tunnel: "Set VDD" -> [w308 _]
      tunnel: [w305 w2179] -> w73
      tunnel: w72 -> [w299 _]
      tunnel: w71 -> [w302 _]
      frame False {
        w345 = u64 0 ("Total Completed")
        w326 = u32 100 ("milliseconds to wait")
        w361 = T7 [enum."Voltage 2", enum."Voltage 3", enum."Voltage 1"] items=["Idle...", "Voltage 1", "Voltage 2", "Voltage 3"]
        w363 = T7 [enum."Voltage 2", enum."Voltage 3", enum."Voltage 1"] items=["Idle...", "Voltage 1", "Voltage 2", "Voltage 3"]
        # "VSA"
        # "HS"
        # "HD/CYC"
        # "DVA"
        # "E-CAL"
        # "VPI"
        # "Verify Socket"
        n92 = for {
          tunnel: w365 -> [w2178]
          tunnel: w364 -> [w2177]
          tunnel: w363 -> [w2175] mode=indexing
          tunnel: [w2171] -> w358
          tunnel: [w2174] -> w348
          tunnel: w308 -> [w2168]
          n93 = call "E3631A_Voltage Controller updated.vi"("VISA resource name"=w2177, "I_VDD(A)"=0.5, "Channel Controller"=w2175, "Voltage 1"=w2168, "Voltage 2"=3.3, "error in (no error)"=w2178, "I_3.3V (A)"=0.5) -> ("VISA resource name out"=w2174:refnum<visa-resource-name>, "error out"=w2172:errorcluster)  [unwired: 7 in]
          n94 = call "Delay.vi"("milliseconds to wait"=u32 100, "error in (no error)"=w2172) -> ("error out"=w2171:errorcluster)  [unwired: 9 in]
        }
        n95 = Array Size(array=w299) -> (size(s)=w301:i32[])
        n96 = Index Array(array=w301) -> (element=w300:i32)  [unwired: 1 in]
        n97 = local write "TTCompleted"(w345) -> ()
        n98 = local write "Total Time"(w345) -> ()
        n99 = for {
          N: w300 -> [_]
          tunnel: w299 -> [w369]
          tunnel: [w368] -> w298 mode=indexing
          i -> [w370]
          n100 = Index Array(array=w369, index (row)=w370, index (col)=0 ("disabled index (col)")) -> (element=w368:dbl)
        }
        "CP to Run" <- w298
        n101 = call "WSVCAP SHL Host TL RFFE Write - Multiple DUTs - Common Data.vi"("Data Out"="074000", "error in"=w358, "Log (T)"=FALSE) -> ("error out"=w359:errorcluster)  [unwired: 12 in]
        n102 = local read "IDD Brd(uA)"() -> (w333:string)
        n103 = call "Delay.vi"("milliseconds to wait"=w326, "error in (no error)"=w359) -> ("error out"=w357:errorcluster)  [unwired: 9 in]
        n104 = call "Ke2000 Single Reading.vi"("error in (no error)"=w357, "VISA resource name"=w356) -> ("error out"=w334:errorcluster, "VISA resource name out"=w355:refnum<visa-resource-name>, "uA"=w336:string)  [unwired: 5 in, 2 out]
        n105 = call "Substration.vi"("error in (no error)"=w334, "Input2"=w333, "Input1"=w336) -> ("error out"=w312:errorcluster, "In1 - In2"=w335:string)  [unwired: 7 in]
        "IDD Stdby(uA)" <- w335
        n106 = case shown="True" w321 {
          tunnel: [1 ("X Repeat") w446] -> w347
          frame False {
          }
          frame True {
            n107 = local read "X Repeat"() -> (w446:i32)
          }
        }
        n108 = call "WSVCAP SHL Host TL RFFE Write - Multiple DUTs - Common Data.vi"("Data Out"="074040", "error in"=w312, "Log (T)"=FALSE) -> ("error out"=w311:errorcluster)  [unwired: 12 in]
        n109 = call "Delay.vi"("milliseconds to wait"=w326, "error in (no error)"=w311) -> ("error out"=w342:errorcluster)  [unwired: 9 in]
        n110 = case shown="True" w319 {
          tunnel: w342 -> [w397 w406]
          tunnel: [w396 w404] -> w340
          tunnel: ["DVA OFF" ("Data Out") "DVA ON" ("Data Out")] -> w341
          frame False {
            n111 = call "WSVCAP SHL Host TL RFFE Write - Multiple DUTs - Common Data.vi"("Data Out"="074820", "error in"=w397) -> ("error out"=w396:errorcluster)  [unwired: 13 in]
          }
          frame True {
            n112 = call "WSVCAP SHL Host TL RFFE Write - Multiple DUTs - Common Data.vi"("Data Out"="074800", "error in"=w406, "Log (T)"=FALSE) -> ("error out"=w402:errorcluster)  [unwired: 12 in]
            n113 = case shown="1" "CP with DVA ON" {
              selector: "CP with DVA ON" -> [w412 w416 w420 w424 w428 w432 w436 w440 w444]
              tunnel: [w411 w415 w419 w423 w427 w431 w435 w439 w442] -> w399
              tunnel: [w410 w414 w418 w422 w426 w430 w434 w438 w443] -> w401
              tunnel: w402 -> [w410 w414 w418 w422 w426 w430 w434 w438 w443]
              tunnel: string[] ["07476F", "074776", "074765", "074769", "07477B", "07477C", "07477D", "074779", "07476B"] -> [w409 w413 w417 w421 w425 w429 w433 w437 w441]
              frame 0, Default {
                n114 = Index Array(array=w409, index=w412) -> (element=w411:string)
              }
              frame 2 {
                n115 = Index Array(array=w413, index=w416) -> (element=w415:string)
              }
              frame 3 {
                n116 = Index Array(array=w417, index=w420) -> (element=w419:string)
              }
              frame 4 {
                n117 = Index Array(array=w421, index=w424) -> (element=w423:string)
              }
              frame 5 {
                n118 = Index Array(array=w425, index=w428) -> (element=w427:string)
              }
              frame 6 {
                n119 = Index Array(array=w429, index=w432) -> (element=w431:string)
              }
              frame 7 {
                n120 = Index Array(array=w433, index=w436) -> (element=w435:string)
              }
              frame 8 {
                n121 = Index Array(array=w437, index=w440) -> (element=w439:string)
              }
              frame 1 {
                n122 = Index Array(array=w441, index=w444) -> (element=w442:string)
              }
            }
            n123 = call "WSVCAP SHL Host TL RFFE Write - Multiple DUTs - Common Data.vi"("Data Out"=w399, "error in"=w401, "Log (T)"=FALSE) -> ("error out"=w404:errorcluster)  [unwired: 12 in]
          }
        }
        n124 = for {
          N: 36 -> [_]
          tunnel: "Serial Number" -> [w379]
          tunnel: [w377] -> w324 mode=indexing
          i -> [w376]
          n125 = Increment(x=w376) -> (x+1=w375:i32)
          n126 = Index Array(array=w379, index (row)=w375, index (col)=1 ("disabled index (col)")) -> (element=w377:string)
        }
        n127 = Not(x=w316) -> (.not. x?=w323:bool)
        n128 = Number To Fractional String(number=w308, precision (6)=i16 2) -> (F-format string=w338:string)  [unwired: 2 in]
        n129 = call "Delay.vi"("milliseconds to wait"=w326, "error in (no error)"=w340) -> ("error out"=w329:errorcluster)  [unwired: 9 in]
        n130 = case shown="True" w320 {
          tunnel: w329 -> [w383 w385]
          tunnel: [w380 w384] -> w328
          tunnel: ["CAL OFF" ("Data Out") "CAL ON" ("Data Out")] -> w330
          frame False {
            n131 = call "WSVCAP SHL Host TL RFFE Write - Multiple DUTs - Common Data.vi"("Data Out"="074044", "error in"=w383) -> ("error out"=w380:errorcluster)  [unwired: 13 in]
          }
          frame True {
            n132 = for {
              tunnel: string[] ["074900", "074920", "074900"] -> [w393] mode=indexing
              tunnel: w385 -> [w390]
              tunnel: [w389] -> w384
              n133 = call "WSVCAP SHL Host TL RFFE Write - Multiple DUTs - Common Data.vi"("Data Out"=w393, "error in"=w390, "Log (T)"=FALSE) -> ("error out"=w392:errorcluster)  [unwired: 12 in]
              n134 = call "Delay.vi"("milliseconds to wait"=u32 10, "error in (no error)"=w392) -> ("error out"=w389:errorcluster)  [unwired: 9 in]
            }
          }
        }
        n135 = for {
          N: w347 -> [_]
          tunnel: w366 -> [w488]
          tunnel: [w487] -> w362
          tunnel: w335 -> [w486]
          tunnel: w355 -> [w485]
          tunnel: "TMN DC\\CAP Data Log File Path" -> [w484]
          tunnel: w353 -> [w483]
          tunnel: [w482] -> w351
          tunnel: w348 -> [w450]
          shift-right: [w477] -> _
          shift-left: u64 0 -> [w479]
          tunnel: w321 -> [w476]
          tunnel: w344 -> [w471]
          tunnel: w344 -> [w470]
          tunnel: w341 -> [w469]
          tunnel: w338 -> [w468]
          tunnel: [w467] -> w332
          tunnel: w330 -> [w466]
          tunnel: w328 -> [w465]
          tunnel: w319 -> [w464]
          tunnel: w322 -> [w463]
          tunnel: w318 -> [w462]
          tunnel: w323 -> [w461]
          tunnel: w317 -> [w460]
          tunnel: w324 -> [w457]
          tunnel: [w449] -> w313
          tunnel: w310 -> [w459]
          tunnel: w309 -> [w458]
          tunnel: "Serial Number" -> [w455]
          tunnel: w299 -> [w452]
          tunnel: [w451] -> w306
          tunnel: w302 -> [w447]
          i -> [w475]
          stop <- w451 stop-if-true
          n136 = while {
            tunnel: w488 -> [w747]
            tunnel: w484 -> [w758]
            tunnel: "Lot#" -> [w757]
            tunnel: "Wafer#" -> [w756]
            tunnel: w457 -> [w755]
            tunnel: "Test Program" -> [w754]
            tunnel: w457 -> [w753]
            tunnel: "Comment" -> [w752]
            tunnel: "Lot#" -> [w751]
            tunnel: "Wafer#" -> [w750]
            tunnel: w485 -> [w746]
            tunnel: [w749] -> w487
            tunnel: w486 -> [w745]
            tunnel: w483 -> [w743]
            tunnel: [w742] -> w482
            tunnel: [w650] -> w473
            tunnel: w475 -> [w688]
            tunnel: [w679] -> w477
            tunnel: w479 -> [w678]
            shift-right: [w677] -> _
            shift-left: u64 0 -> [w574]
            tunnel: [w676] -> w472
            tunnel: w476 -> [w674]
            tunnel: w471 -> [w649]
            tunnel: w470 -> [w647]
            tunnel: w469 -> [w597]
            tunnel: w468 -> [w595]
            tunnel: [w571] -> w467
            tunnel: w466 -> [w578]
            tunnel: w465 -> [w577]
            tunnel: w464 -> [w576]
            tunnel: w463 -> [w568]
            tunnel: w462 -> [w567]
            tunnel: w461 -> [w562]
            tunnel: w460 -> [w556]
            tunnel: w459 -> [w532]
            tunnel: w458 -> [w531]
            tunnel: w455 -> [w516]
            tunnel: "Test Program" -> [w515]
            tunnel: "Lot#" -> [w514]
            tunnel: "Wafer#" -> [w513]
            tunnel: "Comment" -> [w510]
            tunnel: w452 -> [w507]
            tunnel: w450 -> [w501]
            tunnel: [w500] -> w449
            tunnel: w447 -> [w496]
            i -> [w675]
            stop <- w689 stop-if-true
            n137 = case shown="8" "CP to HD/Cycle" {
              selector: "CP to HD/Cycle" -> [w762 w767 w772 w777 w782 w787 w792 w797 w801]
              tunnel: string[] ["07476F", "074776", "074765", "074769", "07477B", "07477C", "07477D", "074779", "07476B"] -> [w763 w768 w773 w778 w783 w788 w793 w798 w803]
              tunnel: [w761 w766 w771 w776 w781 w786 w791 w796 w802] -> w593
              tunnel: ["35.0" ("Data Out") "27.5" ("Data Out") "30.5" ("Data Out") "44.0" ("Data Out") "50.0" ("Data Out") "55.0" ("Data Out") "42.5" ("Data Out") "32.0" ("Data Out") "40.25" ("Data Out")] -> w592
              tunnel: [w759 w764 w769 w774 w779 w784 w789 w794 w799] -> w591
              tunnel: w577 -> [w759 w764 w769 w774 w779 w784 w789 w794 w799]
              frame 0, Default {
                n138 = Index Array(array=w763, index=w762) -> (element=w761:string)
              }
              frame 2 {
                n139 = Index Array(array=w768, index=w767) -> (element=w766:string)
              }
              frame 3 {
                n140 = Index Array(array=w773, index=w772) -> (element=w771:string)
              }
              frame 4 {
                n141 = Index Array(array=w778, index=w777) -> (element=w776:string)
              }
              frame 5 {
                n142 = Index Array(array=w783, index=w782) -> (element=w781:string)
              }
              frame 6 {
                n143 = Index Array(array=w788, index=w787) -> (element=w786:string)
              }
              frame 7 {
                n144 = Index Array(array=w793, index=w792) -> (element=w791:string)
              }
              frame 8 {
                n145 = Index Array(array=w798, index=w797) -> (element=w796:string)
              }
              frame 1 {
                n146 = Index Array(array=w803, index=w801) -> (element=w802:string)
              }
            }
            n147 = flat-sequence {
              tunnel: [w871] -> w741
              tunnel: [w866] -> w740
              tunnel: w747 -> [w869]
              tunnel: [w868] -> w739
              tunnel: w746 -> [w846]
              tunnel: w745 -> [w867]
              tunnel: [w867] -> w738
              tunnel: [w819] -> w737
              tunnel: [w816] -> w736
              tunnel: w591 -> [w859]
              tunnel: w688 -> [w864]
              tunnel: w675 -> [w842]
              tunnel: [w842] -> w685
              tunnel: w675 -> [w863]
              tunnel: w674 -> [w861]
              tunnel: [w860] -> w673
              tunnel: [w825] -> w668
              tunnel: [w824] -> w667
              tunnel: [w823] -> w666
              tunnel: [w829] -> w656
              tunnel: [w826] -> w655
              tunnel: w649 -> [w858]
              tunnel: [w858] -> w648
              tunnel: w647 -> [w857]
              tunnel: [w828] -> w635
              tunnel: [w827] -> w610
              tunnel: [w856] -> w598
              tunnel: w593 -> [w854]
              tunnel: [w843] -> w590
              tunnel: [w809] -> w582
              tunnel: w568 -> [w839]
              tunnel: w567 -> [w838]
              tunnel: [w838] -> w566
              tunnel: w562 -> [w837]
              tunnel: [w837] -> w561
              tunnel: w556 -> [w836]
              tunnel: [w836] -> w555
              tunnel: [w832] -> w550
              tunnel: ["Test Sequences"] -> w546
              tunnel: "Real No. From\nLookup Table" -> [w822]
              tunnel: ["WS1050/51"] -> w540
              tunnel: ["Cmin/Act"] -> w536
              tunnel: w532 -> [w811]
              tunnel: w531 -> [w810]
              tunnel: w741 -> [w1180]
              tunnel: w740 -> [w1205]
              tunnel: w739 -> [w1210]
              tunnel: [w1210] -> w646
              tunnel: w738 -> [w1209]
              tunnel: w737 -> [w1204]
              tunnel: w736 -> [w1203]
              tunnel: [w1194] -> w645
              tunnel: [w1209] -> w644
              tunnel: [w1204] -> w643
              tunnel: [w1203] -> w642
              tunnel: w685 -> [w1207]
              tunnel: [w1207] -> w641
              tunnel: w673 -> [w1206]
              tunnel: [w1206] -> w640
              tunnel: [w1205] -> w639
              tunnel: w668 -> [w1202]
              tunnel: w667 -> [w1187]
              tunnel: w666 -> [w1188]
              tunnel: [w1199] -> w638
              tunnel: w656 -> [w1201]
              tunnel: w655 -> [w1199]
              tunnel: [w1195] -> w637
              tunnel: w648 -> [w1200]
              tunnel: [w1185] -> w636
              tunnel: w635 -> [w1185]
              tunnel: [w1187] -> w634
              tunnel: w610 -> [w1186]
              tunnel: [w1186] -> w609
              tunnel: [w1188] -> w607
              tunnel: w598 -> [w1198]
              tunnel: [w1197] -> w583
              tunnel: w582 -> [w1197]
              tunnel: w566 -> [w1193]
              tunnel: [w1193] -> w565
              tunnel: w561 -> [w1192]
              tunnel: [w1192] -> w560
              tunnel: w555 -> [w1191]
              tunnel: [w1191] -> w554
              tunnel: w550 -> [w1190]
              tunnel: [w1189] -> w549
              tunnel: w546 -> [w1183]
              tunnel: [w1183] -> w545
              tunnel: w540 -> [w1182]
              tunnel: [w1182] -> w539
              tunnel: w536 -> [w1181]
              tunnel: [w1181] -> w535
              tunnel: [w1180] -> w529
              tunnel: w646 -> [w1333]
              tunnel: [w1333] -> w631
              tunnel: w645 -> [w1315]
              tunnel: [w1315] -> w629
              tunnel: w644 -> [w1332]
              tunnel: [w1332] -> w627
              tunnel: w643 -> [w1331]
              tunnel: [w1331] -> w625
              tunnel: w642 -> [w1330]
              tunnel: [w1330] -> w623
              tunnel: w641 -> [w1329]
              tunnel: [w1329] -> w621
              tunnel: w640 -> [w1328]
              tunnel: [w1328] -> w619
              tunnel: w639 -> [w1327]
              tunnel: [w1327] -> w617
              tunnel: w638 -> [w1326]
              tunnel: [w1326] -> w615
              tunnel: [w1320] -> w613
              tunnel: w637 -> [w1319]
              tunnel: w636 -> [w1324]
              tunnel: w634 -> [w1323]
              tunnel: w609 -> [w1312]
              tunnel: [w1312] -> w608
              tunnel: w607 -> [w1314]
              tunnel: [w1314] -> w606
              tunnel: [w1321] -> w605
              tunnel: [w1322] -> w584
              tunnel: w583 -> [w1322]
              tunnel: w565 -> [w1318]
              tunnel: [w1318] -> w564
              tunnel: w560 -> [w1317]
              tunnel: [w1317] -> w559
              tunnel: w554 -> [w1316]
              tunnel: [w1316] -> w553
              tunnel: w549 -> [w1313]
              tunnel: w545 -> [w1310]
              tunnel: [w1313] -> w544
              tunnel: [w1310] -> w543
              tunnel: w539 -> [w1309]
              tunnel: [w1309] -> w538
              tunnel: w535 -> [w1308]
              tunnel: [w1308] -> w534
              tunnel: w529 -> [w1307]
              tunnel: [w1307] -> w528
              tunnel: w496 -> [w1306]
              tunnel: [w1306] -> w495
              tunnel: [w1401] -> w633
              tunnel: [w1413] -> w632
              tunnel: w631 -> [w1428]
              tunnel: [w1428] -> w630
              tunnel: w629 -> [w1407]
              tunnel: [w1407] -> w628
              tunnel: w627 -> [w1427]
              tunnel: [w1427] -> w626
              tunnel: w625 -> [w1426]
              tunnel: [w1426] -> w624
              tunnel: w623 -> [w1425]
              tunnel: [w1425] -> w622
              tunnel: w621 -> [w1424]
              tunnel: [w1424] -> w620
              tunnel: w619 -> [w1423]
              tunnel: [w1423] -> w618
              tunnel: w617 -> [w1422]
              tunnel: [w1422] -> w616
              tunnel: w615 -> [w1421]
              tunnel: [w1421] -> w614
              tunnel: w613 -> [w1420]
              tunnel: [w1420] -> w612
              tunnel: [w1404] -> w611
              tunnel: w608 -> [w1418]
              tunnel: w606 -> [w1417]
              tunnel: w605 -> [w1412]
              tunnel: ["DeltaC Target Setting(pF)"] -> w596
              tunnel: [w1415] -> w585
              tunnel: w584 -> [w1415]
              tunnel: w576 -> [w1414]
              tunnel: [w1414] -> w575
              tunnel: w564 -> [w1411]
              tunnel: [w1411] -> w563
              tunnel: w559 -> [w1410]
              tunnel: [w1410] -> w558
              tunnel: w553 -> [w1409]
              tunnel: [w1409] -> w552
              tunnel: w544 -> [w1408]
              tunnel: w543 -> [w1405]
              tunnel: [w1404] -> w541
              tunnel: w538 -> [w1403]
              tunnel: [w1403] -> w537
              tunnel: w534 -> [w1402]
              tunnel: [w1402] -> w533
              tunnel: w528 -> [w1401]
              tunnel: w495 -> [w1400]
              tunnel: [w1400] -> w494
              tunnel: [w1496] -> w735
              tunnel: [w1516] -> w734
              tunnel: w633 -> [w1496]
              tunnel: w632 -> [w1530]
              tunnel: [w1539] -> w733
              tunnel: [w1530] -> w732
              tunnel: [w1552] -> w731
              tunnel: [w1551] -> w730
              tunnel: w630 -> [w1550]
              tunnel: [w1550] -> w729
              tunnel: w628 -> [w1539]
              tunnel: w626 -> [w1549]
              tunnel: [w1549] -> w728
              tunnel: w624 -> [w1545]
              tunnel: [w1545] -> w727
              tunnel: w622 -> [w1544]
              tunnel: [w1544] -> w726
              tunnel: w620 -> [w1540]
              tunnel: [w1540] -> w684
              tunnel: w618 -> [w1548]
              tunnel: [w1548] -> w672
              tunnel: w616 -> [w1547]
              tunnel: [w1546] -> w669
              tunnel: w614 -> [w1542]
              tunnel: w612 -> [w1538]
              tunnel: [w1543] -> w665
              tunnel: [w1541] -> w664
              tunnel: [w1538] -> w659
              tunnel: w611 -> [w1537]
              tunnel: [w1524] -> w654
              tunnel: [w1523] -> w653
              tunnel: [w1522] -> w652
              tunnel: w596 -> [w1536]
              tunnel: [w1521] -> w586
              tunnel: w585 -> [w1521]
              tunnel: [w1520] -> w581
              tunnel: w575 -> [w1519]
              tunnel: w563 -> [w1514]
              tunnel: w558 -> [w1513]
              tunnel: [w1513] -> w557
              tunnel: w552 -> [w1512]
              tunnel: [w1512] -> w551
              tunnel: w541 -> [w1509]
              tunnel: w537 -> [w1508]
              tunnel: w533 -> [w1497]
              tunnel: w494 -> [w1495]
              tunnel: [w1495] -> w493
              tunnel: w735 -> [w1748]
              tunnel: [w1748] -> w725
              tunnel: [w1775] -> w724
              tunnel: [w1789] -> w723
              tunnel: w734 -> [w1788]
              tunnel: w733 -> [w1787]
              tunnel: w732 -> [w1786]
              tunnel: [w1787] -> w722
              tunnel: [w1786] -> w721
              tunnel: w731 -> [w1785]
              tunnel: [w1785] -> w720
              tunnel: w730 -> [w1784]
              tunnel: [w1784] -> w719
              tunnel: w729 -> [w1783]
              tunnel: [w1783] -> w718
              tunnel: w728 -> [w1782]
              tunnel: [w1782] -> w717
              tunnel: w727 -> [w1781]
              tunnel: [w1781] -> w716
              tunnel: w726 -> [w1780]
              tunnel: [w1780] -> w715
              tunnel: w743 -> [w1779]
              tunnel: [w1777] -> w714
              tunnel: [w1757] -> w713
              tunnel: [w1758] -> w712
              tunnel: [w1756] -> w711
              tunnel: w684 -> [w1773]
              tunnel: [w1773] -> w683
              tunnel: w672 -> [w1772]
              tunnel: [w1772] -> w671
              tunnel: w669 -> [w1789]
              tunnel: w665 -> [w1770]
              tunnel: w664 -> [w1771]
              tunnel: [w1771] -> w663
              tunnel: [w1770] -> w661
              tunnel: w659 -> [w1769]
              tunnel: [w1769] -> w658
              tunnel: w654 -> [w1755]
              tunnel: w653 -> [w1754]
              tunnel: w652 -> [w1753]
              tunnel: [w1750] -> w651
              tunnel: [w1755] -> w604
              tunnel: [w1754] -> w602
              tunnel: [w1753] -> w600
              tunnel: [w1752] -> w587
              tunnel: w586 -> [w1752]
              tunnel: w581 -> [w1751]
              tunnel: [w1751] -> w580
              tunnel: w557 -> [w1750]
              tunnel: w551 -> [w1749]
              tunnel: w493 -> [w1747]
              tunnel: [w1747] -> w492
              tunnel: w725 -> [w1898]
              tunnel: [w1898] -> w710
              tunnel: w724 -> [w1922]
              tunnel: [w1921] -> w709
              tunnel: w758 -> [w1923]
              tunnel: w757 -> [w1920]
              tunnel: w756 -> [w1919]
              tunnel: w755 -> [w1918]
              tunnel: [w1917] -> w708
              tunnel: w723 -> [w1911]
              tunnel: [w1911] -> w707
              tunnel: w722 -> [w1916]
              tunnel: w721 -> [w1915]
              tunnel: [w1916] -> w706
              tunnel: [w1915] -> w705
              tunnel: [w1906] -> w704
              tunnel: w720 -> [w1914]
              tunnel: [w1914] -> w703
              tunnel: w719 -> [w1913]
              tunnel: [w1913] -> w702
              tunnel: w718 -> [w1910]
              tunnel: [w1912] -> w701
              tunnel: w574 -> [w1909]
              tunnel: [w1908] -> w700
              tunnel: [w1896] -> w699
              tunnel: w717 -> [w1907]
              tunnel: w716 -> [w1905]
              tunnel: w715 -> [w1904]
              tunnel: "File Name" -> [w1903]
              tunnel: w714 -> [w1902]
              tunnel: [w1902] -> w698
              tunnel: w713 -> [w1901]
              tunnel: [w1901] -> w697
              tunnel: [w1900] -> w696
              tunnel: w712 -> [w1900]
              tunnel: w711 -> [w1899]
              tunnel: [w1899] -> w695
              tunnel: [w1894] -> w686
              tunnel: w683 -> [w1895]
              tunnel: [w1895] -> w681
              tunnel: w678 -> [w1893]
              tunnel: w671 -> [w1892]
              tunnel: [w1892] -> w670
              tunnel: w663 -> [w1891]
              tunnel: [w1891] -> w662
              tunnel: w661 -> [w1890]
              tunnel: [w1890] -> w660
              tunnel: w658 -> [w1889]
              tunnel: [w1889] -> w657
              tunnel: w651 -> [w1888]
              tunnel: w604 -> [w1887]
              tunnel: [w1887] -> w603
              tunnel: w602 -> [w1886]
              tunnel: [w1886] -> w601
              tunnel: w600 -> [w1885]
              tunnel: [w1885] -> w599
              tunnel: w590 -> [w1884]
              tunnel: [w1884] -> w589
              tunnel: [w1883] -> w588
              tunnel: w587 -> [w1883]
              tunnel: w580 -> [w1882]
              tunnel: [w1882] -> w579
              tunnel: ["Freq(Hz)"] -> w548
              tunnel: ["Board#"] -> w547
              tunnel: w492 -> [w1879]
              tunnel: [w1879] -> w491
              tunnel: w710 -> [w1949]
              tunnel: w709 -> [w1997]
              tunnel: w758 -> [w1947]
              tunnel: w754 -> [w1992]
              tunnel: w753 -> [w1995]
              tunnel: w752 -> [w1991]
              tunnel: w751 -> [w1994]
              tunnel: w750 -> [w1990]
              tunnel: w708 -> [w1993]
              tunnel: [w1949] -> w691
              tunnel: [w1996] -> w692
              tunnel: w707 -> [w1989]
              tunnel: [w1989] -> w693
              tunnel: w706 -> [w1988]
              tunnel: w705 -> [w1974]
              tunnel: w704 -> [w1987]
              tunnel: w703 -> [w1986]
              tunnel: w702 -> [w1976]
              tunnel: [w1983] -> w694
              tunnel: w701 -> [w1985]
              tunnel: w700 -> [w1984]
              tunnel: w699 -> [w1983]
              tunnel: "File Name" -> [w1956]
              tunnel: w698 -> [w1982]
              tunnel: [w1982] -> w690
              tunnel: w697 -> [w1981]
              tunnel: w696 -> [w1980]
              tunnel: w695 -> [w1979]
              tunnel: [w1978] -> w687
              tunnel: w686 -> [w1978]
              tunnel: [w1959] -> w682
              tunnel: w681 -> [w1959]
              tunnel: w670 -> [w1944]
              tunnel: w662 -> [w1977]
              tunnel: w660 -> [w1975]
              tunnel: w657 -> [w1973]
              tunnel: w603 -> [w1972]
              tunnel: w601 -> [w1971]
              tunnel: w599 -> [w1970]
              tunnel: w597 -> [w1969]
              tunnel: w578 -> [w1968]
              tunnel: w592 -> [w1967]
              tunnel: w595 -> [w1966]
              tunnel: w589 -> [w1965]
              tunnel: w588 -> [w1964]
              tunnel: w579 -> [w1963]
              tunnel: [w1961] -> w573
              tunnel: [w1952] -> w569
              tunnel: w548 -> [w1951]
              tunnel: w547 -> [w1946]
              tunnel: [w1947] -> w518
              tunnel: [w1946] -> w512
              tunnel: w510 -> [w1945]
              tunnel: [w1945] -> w509
              tunnel: [w1944] -> w498
              tunnel: w491 -> [w1943]
              tunnel: [w1943] -> w490
              tunnel: w694 -> [w2039]
              tunnel: w693 -> [w2056]
              tunnel: w692 -> [w2045]
              tunnel: w691 -> [w2057]
              tunnel: w690 -> [w2050]
              tunnel: w687 -> [w2048]
              tunnel: w682 -> [w2049]
              tunnel: w573 -> [w2043]
              tunnel: w569 -> [w2041]
              tunnel: [w2057] -> w527
              tunnel: [w2056] -> w526
              tunnel: [w2055] -> w525
              tunnel: [w2050] -> w524
              tunnel: [w2048] -> w523
              tunnel: [w2049] -> w522
              tunnel: [w2039] -> w521
              tunnel: [w2047] -> w520
              tunnel: [w2044] -> w519
              tunnel: w518 -> [w2038]
              tunnel: [w2038] -> w517
              tunnel: w512 -> [w2037]
              tunnel: [w2037] -> w511
              tunnel: w509 -> [w2036]
              tunnel: [w2036] -> w508
              tunnel: w507 -> [w2035]
              tunnel: [w2035] -> w506
              tunnel: w501 -> [w2034]
              tunnel: [w2034] -> w502
              tunnel: ["CP CV \nSweep"] -> w499
              tunnel: w498 -> [w2032]
              tunnel: [w2032] -> w497
              tunnel: w490 -> [w2031]
              tunnel: [w2031] -> w489
              tunnel: [w2093] -> w570
              tunnel: [w2096] -> w676
              tunnel: [w2094] -> w677
              tunnel: [w2097] -> w680
              tunnel: [w2098] -> w679
              tunnel: [w2084] -> w742
              tunnel: [w2099] -> w748
              tunnel: [w2082] -> w749
              tunnel: [w2100] -> w650
              tunnel: w527 -> [w2100]
              tunnel: w526 -> [w2083]
              tunnel: w525 -> [w2099]
              tunnel: w524 -> [w2085]
              tunnel: w523 -> [w2098]
              tunnel: w522 -> [w2097]
              tunnel: w521 -> [w2094]
              tunnel: w520 -> [w2096]
              tunnel: w519 -> [w2095]
              tunnel: w517 -> [w2092]
              tunnel: w516 -> [w2091]
              tunnel: w515 -> [w2090]
              tunnel: w514 -> [w2089]
              tunnel: w513 -> [w2088]
              tunnel: w511 -> [w2087]
              tunnel: w508 -> [w2077]
              tunnel: w506 -> [w2076]
              tunnel: w503 -> [w2086]
              tunnel: w502 -> [w2081]
              tunnel: [w2080] -> w500
              tunnel: w499 -> [w2079]
              tunnel: w497 -> [w2078]
              tunnel: w489 -> [w2075]
              frame #0 {
                w833 = FALSE ("Log (T)")
                n148 = call "WSVCAP SHL Host TL RFFE Write - Multiple DUTs - Common Data.vi"("Data Out"=w854, "error in"=w859, "Log (T)"=FALSE) -> ("error out"=w840:errorcluster)  [unwired: 12 in]
                n149 = Index Array(array=w869, index (row)=w863, index (col)=0 ("disabled index (col)")) -> (element=w862:dbl)
                n150 = for {
                  tunnel: string[] ["0760", "0767", "0768"] -> [w938] mode=indexing
                  tunnel: [w934] -> w844 mode=indexing
                  tunnel: w840 -> [w932]
                  tunnel: [w931] -> w841
                  i -> [w937]
                  n151 = call "Delay.vi"("milliseconds to wait"=u32 10, "error in (no error)"=w932) -> ("error out"=w939:errorcluster)  [unwired: 9 in]
                  n152 = call "WSVCAP SHL Host TL RFFE Read - Multiple DUTs - Common Data.vi"("Data Out"=w938, "error in"=w939, "Log (T)"=FALSE) -> ("RFFE Data In"=w936:string[], "error out"=w931:errorcluster)  [unwired: 11 in]
                  n153 = Index Array(array=w936, index=w937) -> (element=w933:string)
                  n154 = String Subset(string=w933, offset (0)=0) -> (substring=w934:string)  [unwired: 1 in]
                }
                "RB Reg for HD/Cycle" <- w844
                n155 = local read "IDD Brd(uA)"() -> (w853:string)
                n156 = call "Delay.vi"("milliseconds to wait"=u32 100, "error in (no error)"=w841) -> ("error out"=w849:errorcluster)  [unwired: 9 in]
                n157 = call "Ke2000 Single Reading.vi"("error in (no error)"=w849, "VISA resource name"=w846) -> ("error out"=w851:errorcluster, "VISA resource name out"=w821:refnum<visa-resource-name>, "uA"=w852:string)  [unwired: 5 in, 2 out]
                n158 = call "Substration.vi"("error in (no error)"=w851, "Input2"=w853, "Input1"=w852) -> ("error out"=w848:errorcluster, "In1 - In2"=→"IDD_HD/CYC (uA)":string)  [unwired: 7 in]
                n159 = case shown="True" w861 {
                  tunnel: [w970 w1075] -> w871
                  tunnel: [w971 w1060] -> w807
                  tunnel: [w969 w1076] -> w868
                  tunnel: w848 -> [w965 w1064]
                  tunnel: w864 -> [_ w1066]
                  tunnel: w862 -> [w962 w1061]
                  tunnel: [w967 w1062] -> w860
                  tunnel: w842 -> [w954 w1058]
                  tunnel: w857 -> [w964 _]
                  tunnel: ["% Duty Cycle" "100" ("Data Out")] -> w843
                  tunnel: w839 -> [w952 _]
                  tunnel: w822 -> [w951 w1053]
                  tunnel: w811 -> [w948 _]
                  tunnel: w810 -> [w947 _]
                  frame False {
                    # "Cycles in 1s"
                    n160 = case shown="True" w951 {
                      tunnel: w965 -> [w977 w983]
                      tunnel: w962 -> [w976 w982]
                      tunnel: [w975 w983] -> w961
                      tunnel: w954 -> [w974 _]
                      tunnel: [w973 w982] -> w960
                      tunnel: [u64 1000 ("y") u64 1 ("y")] -> w955
                      frame False {
                        n161 = case shown="8, Default" w974 {
                          tunnel: w976 -> [w979 _]
                          tunnel: [w979 "Cycle RP"] -> w973
                          tunnel: [w978 w980] -> w975
                          tunnel: w977 -> [w978 w980]
                          frame 0..7 {
                          }
                          frame 8, Default {
                          }
                        }
                      }
                      frame True {
                        # "Read real number\nfrom lookup table"
                      }
                    }
                    n162 = call "WSVCAP SHL Host TL RFFE Configure.vi"("RFFE Slave Address"=w964, "Clock Rate (Hz)"="SPI Clock Rate (Hz)", "error in"=w961) -> ("Actual Rate (Hz)"=→"AR Cycling(Hz)":dbl, "error out"=w950:errorcluster)  [unwired: 11 in]
                    n163 = Array Max & Min(array=w947) -> (max value=w958:dbl)  [unwired: 3 out]
                    n164 = Divide(x=1.0, y=w958) -> (x/y=w957:dbl)
                    n165 = To Unsigned Quad Integer(1:w957) -> (0:w956:u64)
                    n166 = Not(x=w952) -> (.not. x?=w953:bool)
                    n167 = case shown="True" w953 {
                      tunnel: [w986 w1008] -> w971
                      tunnel: [w989 w1007] -> w970
                      tunnel: [u64 1 w1006] -> w969
                      tunnel: w950 -> [w987 w1005]
                      tunnel: w960 -> [_ w1004]
                      tunnel: w947 -> [_ w1002]
                      tunnel: w956 -> [_ w1001]
                      tunnel: w955 -> [_ w1000]
                      tunnel: w954 -> [w985 _]
                      tunnel: w948 -> [_ w999]
                      frame False {
                        n168 = case shown="1, Default" w985 {
                          tunnel: w987 -> [w990 w992]
                          tunnel: [w990 w991] -> w986
                          frame 0 {
                          }
                          frame 1, Default {
                            n169 = flat-sequence {
                              tunnel: "Repeat Meas(s)" -> [w998]
                              tunnel: w992 -> [w995]
                              tunnel: [w995] -> w991
                              frame #0 {
                                n170 = Multiply(x=w998, y=u32 1000) -> (x*y=w997:u32)
                                n171 = Wait (ms)(milliseconds to wait=w997) -> ()  [unwired: 1 out]
                                n172 = local write "STATUS"("Verify Sockets waiting times..." ("STATUS")) -> ()
                              }
                            }
                          }
                        }
                        n173 = local read "stop During HD/Cycles"() -> (w989:bool)
                      }
                      frame True {
                        n174 = while {
                          tunnel: w1004 -> [w1028]
                          tunnel: [w1015] -> w1008
                          tunnel: [w1020] -> w1007
                          tunnel: w1005 -> [w1026]
                          tunnel: [w1014] -> w1006
                          tunnel: w999 -> [w1025]
                          tunnel: w1002 -> [w1024]
                          tunnel: w1001 -> [w1011]
                          tunnel: w1000 -> [w1009]
                          i -> [w1023]
                          stop <- w1019 stop-if-true
                          # "At least 1 second before target"
                          # "Remaining Cycles"
                          # "Target Cycles"
                          # "Cycles in 1s"
                          n175 = To Unsigned Quad Integer(1:w1028) -> (0:w1027:u64)
                          n176 = case shown="0" w1023 {
                            tunnel: [w1036 w1038] -> w1017
                            tunnel: w1026 -> [w1037 w1038]
                            tunnel: w1025 -> [w1035 _]
                            tunnel: w1024 -> [w1034 _]
                            frame 0 {
                              n177 = call "WSVCAP SHL Host TL RFFE Write Cycle - Multiple DUTs - Common Data.vi"("Data Out (Cycle Commands)"=w1035, "Post Command Delay"=w1034, "error in"=w1037, "Log (T)"=FALSE) -> ("error out"=w1036:errorcluster)  [unwired: 11 in]
                            }
                            frame 1, Default {
                            }
                          }
                          n178 = Multiply(x=w1027, y=w1009) -> (x*y=w1014:u64)
                          n179 = call "WSVCAP SHL Host TL SPI_RFFE Query Cycle Count.vi"("error in"=w1017) -> ("Cycle Count"=w1013:u64, "error out"=w1022:errorcluster)  [unwired: 13 in]
                          "Cycle Count" <- w1013
                          n180 = Subtract(x=w1014, y=w1013) -> (x-y=w1012:u64)
                          n181 = Greater Or Equal?(x=w1013, y=w1014) -> (x >= y?=w1021:bool)
                          n182 = local read "stop During HD/Cycles"() -> (w1020:bool)
                          n183 = Greater?(x=w1012, y=w1011) -> (0:w1010:bool)
                          n184 = case shown="True" w1021 {
                            tunnel: [w1040 w1043] -> w1016
                            tunnel: w1022 -> [w1040 w1042]
                            tunnel: [FALSE TRUE] -> w1018
                            frame False {
                            }
                            frame True {
                              n185 = call "WSVCAP SHL Host TL SPI Stop Write Cycle.vi"("error in"=w1042) -> ("error out"=w1043:errorcluster)  [unwired: 14 in]
                            }
                          }
                          n186 = Or(x=w1018, y=w1020) -> (x .or. y?=w1019:bool)
                          n187 = case shown="True" w1010 {
                            tunnel: w1016 -> [w1029 w1032]
                            tunnel: [w1029 w1031] -> w1015
                            frame False {
                            }
                            frame True {
                              n188 = call "MISC Wait with Data Flow.vi"("Error In (no error)"=w1032, "Wait Time (500ms)"=u32 50) -> ("Error Out"=w1031:errorcluster)  [unwired: 7 in, 2 out]
                            }
                          }
                        }
                        n189 = local write "STATUS"("Parts are Cycling...." ("STATUS")) -> ()
                      }
                    }
                    n190 = local read "HD/CYC Temp"() -> (w966:i32)
                    n191 = Number To Engineering String(4:w966) -> (0:w967:string)  [unwired: 3 in]
                  }
                  frame True {
                    n192 = case shown="False" w1053 {
                      tunnel: w1066 -> [w1093 _]
                      tunnel: [w1092 w1105] -> w1065
                      tunnel: w1064 -> [w1091 w1106]
                      tunnel: [w1090 w1106] -> w1063
                      tunnel: w1061 -> [w1089 w1105]
                      tunnel: w1058 -> [w1088 _]
                      frame False {
                        n193 = case shown="1, Default" w1093 {
                          tunnel: [w1096 w1103] -> w1092
                          tunnel: w1091 -> [w1098 w1104]
                          tunnel: [w1097 w1104] -> w1090
                          tunnel: w1089 -> [w1095 _]
                          tunnel: w1088 -> [w1094 _]
                          frame 0 {
                            n194 = case shown="15, Default" w1094 {
                              tunnel: [w1099 "HD RP"] -> w1096
                              tunnel: w1098 -> [w1100 w1101]
                              tunnel: [w1100 w1101] -> w1097
                              tunnel: w1095 -> [w1099 _]
                              frame 0..14 {
                              }
                              frame 15, Default {
                              }
                            }
                          }
                          frame 1, Default {
                            n195 = local read "HD RP"() -> (w1103:dbl)
                          }
                        }
                      }
                      frame True {
                      }
                    }
                    n196 = call "WSVCAP SHL Host TL RFFE Write - Multiple DUTs - Common Data.vi"("Data Out"="Cmd To HD", "error in"=w1063, "Log (T)"=FALSE) -> ("error out"=w1049:errorcluster)  [unwired: 12 in]
                    n197 = local read "No of HD/Cycle\nCompleted"() -> (w1067:u64)
                    n198 = call "Delay.vi"("milliseconds to wait"=u32 50, "error in (no error)"=w1049) -> ("error out"=w1046:errorcluster)  [unwired: 9 in]
                    n199 = for {
                      tunnel: string[] ["0761", "0762", "0763"] -> [w1087] mode=indexing
                      tunnel: [w1083] -> w1045 mode=indexing
                      shift-right: [w1080] -> w1071
                      shift-left: w1046 -> [w1086]
                      i -> [w1085]
                      n200 = call "WSVCAP SHL Host TL RFFE Read - Multiple DUTs - Common Data.vi"("Data Out"=w1087, "error in"=w1086, "Log (T)"=FALSE) -> ("RFFE Data In"=w1082:string[], "error out"=w1079:errorcluster)  [unwired: 11 in]
                      n201 = Index Array(array=w1082, index=w1085) -> (element=w1081:string)
                      n202 = call "Delay.vi"("milliseconds to wait"=u32 10, "error in (no error)"=w1079) -> ("error out"=w1080:errorcluster)  [unwired: 9 in]
                      n203 = String Subset(string=w1081, offset (0)=0) -> (substring=w1083:string)  [unwired: 1 in]
                    }
                    "RB Reg for HD" <- w1045
                    n204 = Greater?(x="HD_DC (Min)", y=w1067) -> (0:w1068:bool)
                    n205 = case shown="True" w1068 {
                      tunnel: [_ w1117] -> w1073
                      tunnel: [w1108 w1116] -> w1072
                      tunnel: w1071 -> [w1108 w1115]
                      tunnel: w1065 -> [w1107 w1114]
                      tunnel: [w1107 w1114] -> w1070
                      frame False {
                      }
                      frame True {
                        n206 = Multiply(x=1000.0, y=w1114) -> (x*y=w1112:dbl)
                        n207 = Multiply(x=60.0, y=w1112) -> (x*y=w1110:dbl)
                        n208 = local write "STATUS"("Parts are Holding Down..." ("STATUS")) -> ()
                        n209 = event shown="[0] Timeout" {
                          selector: _ -> [_ _]
                          dyn-events: _ -> [_ _]
                          timeout: w1110 -> [_ _]
                          tunnel: ["stop During HD/Cycles" TRUE ("stop During HD/Cycles")] -> w1117
                          tunnel: w1115 -> [w1118 w1120]
                          tunnel: [w1118 w1120] -> w1116
                          event Timeout {
                            n210 = event-data() -> ()  [unwired: 1 in, 2 out]
                          }
                          event "stop During HD/Cycles": Value Change {
                            n211 = event-data() -> ()  [unwired: 1 in, 2 out]
                          }
                        }
                      }
                    }
                    n212 = Greater Or Equal?(x=w1067, y="HD_DC (Min)") -> (x >= y?=w1074:bool)
                    n213 = To Unsigned Quad Integer(1:w1065) -> (0:w1076:u64)
                    n214 = Add(x="Time All OFF (s)", y="Time All ON (s)") -> (x+y=w1055:u32)
                    n215 = To Double Precision Float(number=w1055) -> (double precision float=w1054:dbl)
                    n216 = Divide(x=w1054, y=60.0) -> (x/y=w1056:dbl)
                    n217 = case shown="False" w1074 {
                      tunnel: [w1124 w1140] -> w1075
                      tunnel: [w1125 w1132] -> w1060
                      tunnel: w1072 -> [w1125 w1139]
                      tunnel: w1073 -> [w1124 w1138]
                      tunnel: w1070 -> [_ w1137]
                      tunnel: [w1123 w1135] -> w1062
                      tunnel: w1056 -> [_ w1129]
                      tunnel: "Time All OFF (s)" -> [_ w1127]
                      tunnel: "Time All ON (s)" -> [_ w1126]
                      frame False {
                        n218 = Number To Engineering String(4:"HD/CYC Temp") -> (0:w1123:string)  [unwired: 3 in]
                      }
                      frame True {
                        n219 = Divide(x=w1137, y=w1129) -> (x/y=w1136:dbl)
                        n220 = call "WSVCAP SHL Host TL RFFE Write - Multiple DUTs - Common Data.vi"("Data Out"="070201000000", "error in"=w1139, "Log (T)"=FALSE) -> ("error out"=w1142:errorcluster)  [unwired: 12 in]
                        n221 = Round To Nearest(number=w1136) -> (nearest integer value=w1131:dbl)
                        n222 = call "Delay.vi"("milliseconds to wait"=u32 50, "error in (no error)"=w1142) -> ("error out"=w1133:errorcluster)  [unwired: 9 in]
                        n223 = To Long Integer(number=w1131) -> (32bit integer=w1130:i32)
                        "No LPs to RP" <- w1130
                        n224 = for {
                          N: w1130 -> [_]
                          tunnel: w1138 -> [w1160]
                          tunnel: [w1159] -> w1140
                          tunnel: w1133 -> [w1149]
                          tunnel: [w1148] -> w1132
                          tunnel: w1127 -> [w1146]
                          tunnel: w1126 -> [w1144]
                          i -> [w1158]
                          stop <- w1159 stop-if-true
                          w1147 = FALSE ("Log (T)")
                          w1145 = u32 1 ("milliseconds to wait")
                          n225 = Increment(x=w1158) -> (x+1=→"LPs Count":i32)
                          n226 = call "WSVCAP SHL Host TL RFFE Write - Multiple DUTs - Common Data.vi"("Data Out"="074776", "error in"=w1149, "Log (T)"=w1147) -> ("error out"=w1166:errorcluster)  [unwired: 12 in]
                          n227 = call "Delay.vi"("milliseconds to wait"=w1145, "error in (no error)"=w1166) -> ("error out"=w1165:errorcluster)  [unwired: 9 in]
                          n228 = local read "CP to HD/Cycle"() -> (w1151:i32)
                          n229 = call "WSVCAP SHL Host TL RFFE Write - Multiple DUTs - Common Data.vi"("Data Out"="070201000000", "error in"=w1152) -> ("error out"=w1162:errorcluster)  [unwired: 13 in]
                          n230 = call "WSVCAP SHL Host TL RFFE Write - Multiple DUTs - Common Data.vi"("Data Out"="0702013B3B3B", "error in"=w1165, "Log (T)"=w1147) -> ("error out"=w1155:errorcluster)  [unwired: 12 in]
                          n231 = call "Delay.vi"("milliseconds to wait"=w1145, "error in (no error)"=w1155) -> ("error out"=w1154:errorcluster)  [unwired: 9 in]
                          n232 = flat-sequence {
                            tunnel: w1162 -> [w1173]
                            tunnel: [w1171] -> w1148
                            tunnel: w1146 -> [w1168]
                            frame #0 {
                              n233 = local write "STATUS"("Now HD OFF Time..." ("STATUS")) -> ()
                              n234 = Multiply(x=w1168, y=u32 1000) -> (x*y=w1170:u32)
                              n235 = call "Delay.vi"("milliseconds to wait"=w1170, "error in (no error)"=w1173) -> ("error out"=w1171:errorcluster)  [unwired: 9 in]
                            }
                          }
                          n236 = Index Array(array=string[] ["07476F", "074776", "074765", "074769", "07477B"], index=w1151) -> (element=w1156:string)
                          n237 = call "WSVCAP SHL Host TL RFFE Write - Multiple DUTs - Common Data.vi"("Data Out"=w1156, "error in"=w1154, "Log (T)"=w1147) -> ("error out"=w1153:errorcluster)  [unwired: 12 in]
                          n238 = flat-sequence {
                            tunnel: [w1178] -> w1152
                            tunnel: w1153 -> [w1175]
                            tunnel: w1144 -> [w1174]
                            frame #0 {
                              n239 = local write "STATUS"("Now HD ON Time..." ("STATUS")) -> ()
                              n240 = Multiply(x=w1174, y=u32 1000) -> (x*y=w1177:u32)
                              n241 = call "Delay.vi"("milliseconds to wait"=w1177, "error in (no error)"=w1175) -> ("error out"=w1178:errorcluster)  [unwired: 9 in]
                            }
                          }
                          n242 = Unbundle By Name(w1148) -> ("status"=w1161:bool)
                          n243 = Or(x=w1161, y=w1160) -> (x .or. y?=w1159:bool)
                        }
                        n244 = Number To Engineering String(4:"DC_Temp") -> (0:w1135:string)  [unwired: 3 in]
                      }
                    }
                  }
                }
                n245 = case shown="0, Default" "CP to Meas" {
                  selector: "CP to Meas" -> [w875 w880 w885 w890 w895 w900 w905 w910 w914]
                  tunnel: string[] ["07476F", "074776", "074765", "074769", "07477B", "07477C", "07477D", "074779", "07476B"] -> [w876 w881 w886 w891 w896 w901 w906 w911 w916]
                  tunnel: [w874 w879 w884 w889 w894 w899 w904 w909 w915] -> w805
                  tunnel: ["35.0" ("Data Out") "27.5" ("Data Out") "30.5" ("Data Out") "44.0" ("Data Out") "50.0" ("Data Out") "55.0" ("Data Out") "42.5" ("Data Out") "32.0" ("Data Out") "40.25" ("Data Out")] -> w809
                  tunnel: [w872 w877 w882 w887 w892 w897 w902 w907 w912] -> w808
                  tunnel: w807 -> [w872 w877 w882 w887 w892 w897 w902 w907 w912]
                  frame 0, Default {
                    n246 = Index Array(array=w876, index=w875) -> (element=w874:string)
                  }
                  frame 2 {
                    n247 = Index Array(array=w881, index=w880) -> (element=w879:string)
                  }
                  frame 3 {
                    n248 = Index Array(array=w886, index=w885) -> (element=w884:string)
                  }
                  frame 4 {
                    n249 = Index Array(array=w891, index=w890) -> (element=w889:string)
                  }
                  frame 5 {
                    n250 = Index Array(array=w896, index=w895) -> (element=w894:string)
                  }
                  frame 6 {
                    n251 = Index Array(array=w901, index=w900) -> (element=w899:string)
                  }
                  frame 7 {
                    n252 = Index Array(array=w906, index=w905) -> (element=w904:string)
                  }
                  frame 8 {
                    n253 = Index Array(array=w911, index=w910) -> (element=w909:string)
                  }
                  frame 1 {
                    n254 = Index Array(array=w916, index=w914) -> (element=w915:string)
                  }
                }
                n255 = flat-sequence {
                  tunnel: w835 -> [w941]
                  tunnel: [w941] -> w831
                  frame #0 {
                    w943 = "0" ("NOM IDD OFF(uA)")
                    w944 = string[] []
                    w945 = string[][] []
                    n256 = To Long Integer(number=0.0 ("No of Loops to RP")) -> (32bit integer=w942:i32)
                    n257 = local write "Total Delta C1(pF)"(w944) -> ()
                    n258 = local write "Total Delta C2(pF)"(w944) -> ()
                    n259 = local write "Total Delta C3(pF)"(w944) -> ()
                    n260 = local write "Current EFuse Read back"(w944) -> ()
                    n261 = local write "RB Reg for HD"(w944) -> ()
                    n262 = local write "RB Reg for HD/Cycle"(w944) -> ()
                    n263 = local write "NOM IDD ON (uA)"(w943) -> ()
                    n264 = local write "NOM IDD OFF(uA)"(w943) -> ()
                    n265 = local write "LPs Count"(w942) -> ()
                    n266 = local write "No LPs to RP"(w942) -> ()
                    n267 = local write "CAP_C3"(w945) -> ()
                    n268 = local write "CAP_C2"(w945) -> ()
                    n269 = local write "CAP_C1"(w945) -> ()
                    n270 = local write "VSA_V3"(w945) -> ()
                    n271 = local write "VSA_V1"(w945) -> ()
                    n272 = local write "VSA_V2"(w945) -> ()
                    n273 = local write "VPI C1"(w945) -> ()
                    n274 = local write "VPI C2"(w945) -> ()
                    n275 = local write "VPI C3"(w945) -> ()
                    n276 = local write "% Delta C"(w945) -> ()
                  }
                }
                n277 = call "WSVCAP SHL Host TL RFFE Write - Multiple DUTs - Common Data.vi"("Data Out"=w805, "error in"=w808, "Log (T)"=w833) -> ("error out"=w855:errorcluster)  [unwired: 12 in]
                n278 = call "Delay.vi"("milliseconds to wait"=u32 50, "error in (no error)"=w855) -> ("error out"=w814:errorcluster)  [unwired: 9 in]
                n279 = for {
                  tunnel: [w929] -> w866
                  tunnel: [w928] -> w835
                  tunnel: w833 -> [w927]
                  tunnel: w821 -> [w926]
                  tunnel: w814 -> [w922]
                  tunnel: string[] ["0702013B3B3B", "070201000000"] -> [w918] mode=indexing
                  tunnel: [w917] -> w817 mode=indexing
                  n280 = call "WSVCAP SHL Host TL RFFE Write - Multiple DUTs - Common Data.vi"("Data Out"=w918, "error in"=w922, "Log (T)"=w927) -> ("error out"=w923:errorcluster)  [unwired: 12 in]
                  n281 = local read "IDD Brd(uA)"() -> (w919:string)
                  n282 = call "Delay.vi"("milliseconds to wait"=u32 100, "error in (no error)"=w923) -> ("error out"=w924:errorcluster)  [unwired: 9 in]
                  n283 = call "Ke2000 Single Reading.vi"("error in (no error)"=w924, "VISA resource name"=w926) -> ("error out"=w921:errorcluster, "VISA resource name out"=w929:refnum<visa-resource-name>, "uA"=w920:string)  [unwired: 5 in, 2 out]
                  n284 = call "Substration.vi"("error in (no error)"=w921, "Input2"=w919, "Input1"=w920) -> ("error out"=w928:errorcluster, "In1 - In2"=w917:string)  [unwired: 7 in]
                }
                n285 = Index Array(array=w817, index=1) -> (element=w816:string)
                n286 = Index Array(array=w817, index=0) -> (element=w819:string)
                n287 = local read "Clock Rate (Hz)"() -> (w856:dbl)
                n288 = call "Multi Dut Cmd_Header Setting.vi"("WS1050/51"="WS1050/51", "Cmin/Act"="Cmin/Act", "Test Seq"="Test Sequences", "error in (no error)"=w831) -> ("Name 1"=w829:string[], "Name 2"=w828:string[], "Name Header"=w826:string[], "Name 3"=w827:string[], "Cmd 3"=w823:string[], "Cmd 1"=w825:string[], "Cmd 2"=w824:string[], "error out"=w832:errorcluster)  [unwired: 2 in, 2 out]
              }
              frame #1 {
                w1189 = FALSE ("Log (T)")
                n289 = call "WSVCAP SHL Host TL RFFE Configure.vi"("RFFE Slave Address"=w1200, "Clock Rate (Hz)"=w1198, "error in"=w1190) -> ("Actual Rate (Hz)"=w1208:dbl, "error out"=w1196:errorcluster)  [unwired: 11 in]
                n290 = local write "AR  Measurent(Hz)"(w1208) -> ()
                n291 = Array Size(array=w1201) -> (size(s)=w1211:i32)
                n292 = case shown="False" w1180 {
                  tunnel: w1211 -> [w1219 _]
                  tunnel: w1202 -> [w1218 _]
                  tunnel: w1201 -> [w1217 _]
                  tunnel: w1196 -> [w1216 w1305]
                  tunnel: [w1215 w1305] -> w1195
                  tunnel: w1189 -> [w1214 _]
                  tunnel: [w1213 string[][] []] -> w1184
                  tunnel: w1183 -> [w1212 _]
                  frame False {
                    n293 = case shown="0, Default" w1212 {
                      tunnel: w1219 -> [w1226 w1254 w1282]
                      tunnel: w1218 -> [w1225 w1253 w1281]
                      tunnel: w1217 -> [w1224 w1252 w1280]
                      tunnel: w1216 -> [w1223 w1251 w1279]
                      tunnel: [w1222 w1250 w1278] -> w1215
                      tunnel: w1214 -> [w1221 w1249 w1277]
                      tunnel: [w1220 w1248 w1276] -> w1213
                      frame 0, Default {
                        n294 = for {
                          N: w1226 -> [_]
                          tunnel: w1225 -> [w1243]
                          tunnel: [w1239] -> w1220 mode=indexing
                          tunnel: w1224 -> [w1241]
                          tunnel: w1223 -> [w1229]
                          tunnel: [w1231] -> w1222
                          tunnel: w1221 -> [w1230]
                          i -> [w1238]
                          stop <- w1227 stop-if-true
                          n295 = Index Array(array=w1243, index=w1238) -> (element=w1242:string)
                          n296 = Index Array(array=w1241, index=w1238) -> (element=w1240:string)
                          n297 = local write "STATUS"(w1240) -> ()
                          n298 = call "WSVCAP SHL Host TL RFFE Write - Multiple DUTs - Common Data.vi"("Data Out"=w1242, "error in"=w1229, "Log (T)"=FALSE) -> ("error out"=w1233:errorcluster)  [unwired: 12 in]
                          n299 = call "Delay.vi"("milliseconds to wait"=u32 10, "error in (no error)"=w1233) -> ("error out"=w1237:errorcluster)  [unwired: 9 in]
                          n300 = call "WS1050 AD7747 READ 36 DUT.vi"("error in"=w1237, "Log (T)"=w1230, "DUT Mask Mode (All)"=WSVCAP_SHL_I2C_DUT_Mask_Mode_Enum."C1") -> ("error out"=w1235:errorcluster, "AD7747 Values"=w1236:string[][])  [unwired: 7 in]
                          n301 = for {
                            tunnel: w1236 -> [w1246] mode=indexing
                            tunnel: w1235 -> [w1247]
                            tunnel: [w1247] -> w1231
                            tunnel: [w1244] -> w1239 mode=indexing
                            n302 = Index Array(array=w1246, index=1) -> (element=w1244:string)
                          }
                          n303 = Unbundle By Name(w1231) -> ("status"=w1227:bool)
                        }
                      }
                      frame 1 {
                        n304 = for {
                          N: w1254 -> [_]
                          tunnel: w1253 -> [w1271]
                          tunnel: [w1267] -> w1248 mode=indexing
                          tunnel: w1252 -> [w1269]
                          tunnel: w1251 -> [w1257]
                          tunnel: [w1259] -> w1250
                          tunnel: w1249 -> [w1258]
                          i -> [w1266]
                          stop <- w1255 stop-if-true
                          n305 = Index Array(array=w1271, index=w1266) -> (element=w1270:string)
                          n306 = Index Array(array=w1269, index=w1266) -> (element=w1268:string)
                          n307 = local write "STATUS"(w1268) -> ()
                          n308 = call "WSVCAP SHL Host TL RFFE Write - Multiple DUTs - Common Data.vi"("Data Out"=w1270, "error in"=w1257, "Log (T)"=FALSE) -> ("error out"=w1261:errorcluster)  [unwired: 12 in]
                          n309 = call "Delay.vi"("milliseconds to wait"=u32 10, "error in (no error)"=w1261) -> ("error out"=w1265:errorcluster)  [unwired: 9 in]
                          n310 = call "WS1050 AD7747 READ 36 DUT.vi"("error in"=w1265, "Log (T)"=w1258, "DUT Mask Mode (All)"=WSVCAP_SHL_I2C_DUT_Mask_Mode_Enum."C2") -> ("error out"=w1263:errorcluster, "AD7747 Values"=w1264:string[][])  [unwired: 7 in]
                          n311 = for {
                            tunnel: w1264 -> [w1274] mode=indexing
                            tunnel: w1263 -> [w1275]
                            tunnel: [w1275] -> w1259
                            tunnel: [w1272] -> w1267 mode=indexing
                            n312 = Index Array(array=w1274, index=3) -> (element=w1272:string)
                          }
                          n313 = Unbundle By Name(w1259) -> ("status"=w1255:bool)
                        }
                      }
                      frame 2 {
                        n314 = for {
                          N: w1282 -> [_]
                          tunnel: w1281 -> [w1299]
                          tunnel: [w1295] -> w1276 mode=indexing
                          tunnel: w1280 -> [w1297]
                          tunnel: w1279 -> [w1285]
                          tunnel: [w1287] -> w1278
                          tunnel: w1277 -> [w1286]
                          i -> [w1294]
                          stop <- w1283 stop-if-true
                          n315 = Index Array(array=w1299, index=w1294) -> (element=w1298:string)
                          n316 = Index Array(array=w1297, index=w1294) -> (element=w1296:string)
                          n317 = local write "STATUS"(w1296) -> ()
                          n318 = call "WSVCAP SHL Host TL RFFE Write - Multiple DUTs - Common Data.vi"("Data Out"=w1298, "error in"=w1285, "Log (T)"=FALSE) -> ("error out"=w1289:errorcluster)  [unwired: 12 in]
                          n319 = call "Delay.vi"("milliseconds to wait"=u32 10, "error in (no error)"=w1289) -> ("error out"=w1293:errorcluster)  [unwired: 9 in]
                          n320 = call "WS1050 AD7747 READ 36 DUT.vi"("error in"=w1293, "Log (T)"=w1286, "DUT Mask Mode (All)"=WSVCAP_SHL_I2C_DUT_Mask_Mode_Enum."C3") -> ("error out"=w1291:errorcluster, "AD7747 Values"=w1292:string[][])  [unwired: 7 in]
                          n321 = for {
                            tunnel: w1292 -> [w1302] mode=indexing
                            tunnel: w1291 -> [w1303]
                            tunnel: [w1303] -> w1287
                            tunnel: [w1300] -> w1295 mode=indexing
                            n322 = Index Array(array=w1302, index=5) -> (element=w1300:string)
                          }
                          n323 = Unbundle By Name(w1287) -> ("status"=w1283:bool)
                        }
                      }
                    }
                  }
                  frame True {
                  }
                }
                n324 = Transpose 2D Array(2D array=w1184) -> (transposed array=w1194:string[][])
                "CAP_C1" <- w1194
                "NOM IDD ON (uA)" <- w1204
                "NOM IDD OFF(uA)" <- w1203
              }
              frame #2 {
                n325 = Array Size(array=w1324) -> (size(s)=w1325:i32)
                n326 = case shown="True" w1307 {
                  tunnel: w1325 -> [w1341 _]
                  tunnel: w1324 -> [w1340 _]
                  tunnel: w1323 -> [w1339 _]
                  tunnel: [w1338 w1399] -> w1321
                  tunnel: w1319 -> [w1337 w1399]
                  tunnel: w1313 -> [w1336 _]
                  tunnel: [w1335 string[][] []] -> w1311
                  tunnel: w1310 -> [w1334 _]
                  frame False {
                    n327 = case shown="0, 2, Default" w1334 {
                      tunnel: w1341 -> [w1348 w1376]
                      tunnel: w1340 -> [w1347 w1375]
                      tunnel: w1339 -> [w1346 w1374]
                      tunnel: [w1345 w1373] -> w1338
                      tunnel: w1337 -> [w1344 w1372]
                      tunnel: w1336 -> [w1343 w1371]
                      tunnel: [w1342 w1370] -> w1335
                      frame 0, 2, Default {
                        n328 = for {
                          N: w1348 -> [_]
                          tunnel: w1346 -> [w1365]
                          tunnel: [w1361] -> w1342 mode=indexing
                          tunnel: w1347 -> [w1363]
                          tunnel: w1344 -> [w1351]
                          tunnel: [w1353] -> w1345
                          tunnel: w1343 -> [w1352]
                          i -> [w1360]
                          stop <- w1349 stop-if-true
                          n329 = Index Array(array=w1365, index=w1360) -> (element=w1364:string)
                          n330 = Index Array(array=w1363, index=w1360) -> (element=w1362:string)
                          n331 = call "WSVCAP SHL Host TL RFFE Write - Multiple DUTs - Common Data.vi"("Data Out"=w1364, "error in"=w1351, "Log (T)"=FALSE) -> ("error out"=w1355:errorcluster)  [unwired: 12 in]
                          n332 = local write "STATUS"(w1362) -> ()
                          n333 = call "Delay.vi"("milliseconds to wait"=u32 10, "error in (no error)"=w1355) -> ("error out"=w1359:errorcluster)  [unwired: 9 in]
                          n334 = call "WS1050 AD7747 READ 36 DUT.vi"("error in"=w1359, "Log (T)"=w1352, "DUT Mask Mode (All)"=WSVCAP_SHL_I2C_DUT_Mask_Mode_Enum."C2") -> ("error out"=w1357:errorcluster, "AD7747 Values"=w1358:string[][])  [unwired: 7 in]
                          n335 = for {
                            tunnel: w1358 -> [w1368] mode=indexing
                            tunnel: w1357 -> [w1369]
                            tunnel: [w1369] -> w1353
                            tunnel: [w1366] -> w1361 mode=indexing
                            n336 = Index Array(array=w1368, index=3) -> (element=w1366:string)
                          }
                          n337 = Unbundle By Name(w1353) -> ("status"=w1349:bool)
                        }
                      }
                      frame 1 {
                        n338 = for {
                          N: w1376 -> [_]
                          tunnel: w1374 -> [w1393]
                          tunnel: [w1389] -> w1370 mode=indexing
                          tunnel: w1375 -> [w1391]
                          tunnel: w1372 -> [w1379]
                          tunnel: [w1381] -> w1373
                          tunnel: w1371 -> [w1380]
                          i -> [w1388]
                          stop <- w1377 stop-if-true
                          n339 = Index Array(array=w1393, index=w1388) -> (element=w1392:string)
                          n340 = Index Array(array=w1391, index=w1388) -> (element=w1390:string)
                          n341 = call "WSVCAP SHL Host TL RFFE Write - Multiple DUTs - Common Data.vi"("Data Out"=w1392, "error in"=w1379, "Log (T)"=FALSE) -> ("error out"=w1383:errorcluster)  [unwired: 12 in]
                          n342 = local write "STATUS"(w1390) -> ()
                          n343 = call "Delay.vi"("milliseconds to wait"=u32 10, "error in (no error)"=w1383) -> ("error out"=w1387:errorcluster)  [unwired: 9 in]
                          n344 = call "WS1050 AD7747 READ 36 DUT.vi"("error in"=w1387, "Log (T)"=w1380, "DUT Mask Mode (All)"=WSVCAP_SHL_I2C_DUT_Mask_Mode_Enum."C1") -> ("error out"=w1385:errorcluster, "AD7747 Values"=w1386:string[][])  [unwired: 7 in]
                          n345 = for {
                            tunnel: w1386 -> [w1396] mode=indexing
                            tunnel: w1385 -> [w1397]
                            tunnel: [w1397] -> w1381
                            tunnel: [w1394] -> w1389 mode=indexing
                            n346 = Index Array(array=w1396, index=1) -> (element=w1394:string)
                          }
                          n347 = Unbundle By Name(w1381) -> ("status"=w1377:bool)
                        }
                      }
                    }
                  }
                  frame True {
                  }
                }
                n348 = Transpose 2D Array(2D array=w1311) -> (transposed array=w1320:string[][])
                "CAP_C2" <- w1320
              }
              frame #3 {
                n349 = Array Size(array=w1418) -> (size(s)=w1419:i32)
                n350 = case shown="True" w1401 {
                  tunnel: w1419 -> [w1436 _]
                  tunnel: w1418 -> [w1435 _]
                  tunnel: w1417 -> [w1434 _]
                  tunnel: w1412 -> [w1433 w1494]
                  tunnel: w1408 -> [w1432 _]
                  tunnel: [w1431 string[][] []] -> w1406
                  tunnel: w1405 -> [w1430 _]
                  tunnel: [w1429 w1494] -> w1404
                  frame False {
                    n351 = case shown="2" w1430 {
                      tunnel: w1436 -> [w1443 w1471]
                      tunnel: w1435 -> [w1442 w1470]
                      tunnel: w1434 -> [w1441 w1469]
                      tunnel: w1433 -> [w1440 w1468]
                      tunnel: [w1439 w1467] -> w1429
                      tunnel: w1432 -> [w1438 w1466]
                      tunnel: [w1437 w1465] -> w1431
                      frame 0, 1, Default {
                        n352 = for {
                          N: w1443 -> [_]
                          tunnel: w1441 -> [w1460]
                          tunnel: [w1456] -> w1437 mode=indexing
                          tunnel: w1442 -> [w1458]
                          tunnel: w1440 -> [w1446]
                          tunnel: [w1448] -> w1439
                          tunnel: w1438 -> [w1447]
                          i -> [w1455]
                          stop <- w1444 stop-if-true
                          n353 = Index Array(array=w1460, index=w1455) -> (element=w1459:string)
                          n354 = Index Array(array=w1458, index=w1455) -> (element=w1457:string)
                          n355 = local write "STATUS"(w1457) -> ()
                          n356 = call "WSVCAP SHL Host TL RFFE Write - Multiple DUTs - Common Data.vi"("Data Out"=w1459, "error in"=w1446, "Log (T)"=FALSE) -> ("error out"=w1450:errorcluster)  [unwired: 12 in]
                          n357 = call "Delay.vi"("milliseconds to wait"=u32 10, "error in (no error)"=w1450) -> ("error out"=w1454:errorcluster)  [unwired: 9 in]
                          n358 = call "WS1050 AD7747 READ 36 DUT.vi"("error in"=w1454, "Log (T)"=w1447, "DUT Mask Mode (All)"=WSVCAP_SHL_I2C_DUT_Mask_Mode_Enum."C3") -> ("error out"=w1452:errorcluster, "AD7747 Values"=w1453:string[][])  [unwired: 7 in]
                          n359 = for {
                            tunnel: w1453 -> [w1463] mode=indexing
                            tunnel: w1452 -> [w1464]
                            tunnel: [w1464] -> w1448
                            tunnel: [w1461] -> w1456 mode=indexing
                            n360 = Index Array(array=w1463, index=5) -> (element=w1461:string)
                          }
                          n361 = Unbundle By Name(w1448) -> ("status"=w1444:bool)
                        }
                      }
                      frame 2 {
                        n362 = for {
                          N: w1471 -> [_]
                          tunnel: w1469 -> [w1488]
                          tunnel: [w1484] -> w1465 mode=indexing
                          tunnel: w1470 -> [w1486]
                          tunnel: w1468 -> [w1474]
                          tunnel: [w1476] -> w1467
                          tunnel: w1466 -> [w1475]
                          i -> [w1483]
                          stop <- w1472 stop-if-true
                          n363 = Index Array(array=w1488, index=w1483) -> (element=w1487:string)
                          n364 = Index Array(array=w1486, index=w1483) -> (element=w1485:string)
                          n365 = local write "STATUS"(w1485) -> ()
                          n366 = call "WSVCAP SHL Host TL RFFE Write - Multiple DUTs - Common Data.vi"("Data Out"=w1487, "error in"=w1474, "Log (T)"=FALSE) -> ("error out"=w1478:errorcluster)  [unwired: 12 in]
                          n367 = call "Delay.vi"("milliseconds to wait"=u32 10, "error in (no error)"=w1478) -> ("error out"=w1482:errorcluster)  [unwired: 9 in]
                          n368 = call "WS1050 AD7747 READ 36 DUT.vi"("error in"=w1482, "Log (T)"=w1475, "DUT Mask Mode (All)"=WSVCAP_SHL_I2C_DUT_Mask_Mode_Enum."C1") -> ("error out"=w1480:errorcluster, "AD7747 Values"=w1481:string[][])  [unwired: 7 in]
                          n369 = for {
                            tunnel: w1481 -> [w1491] mode=indexing
                            tunnel: w1480 -> [w1492]
                            tunnel: [w1492] -> w1476
                            tunnel: [w1489] -> w1484 mode=indexing
                            n370 = Index Array(array=w1491, index=1) -> (element=w1489:string)
                          }
                          n371 = Unbundle By Name(w1476) -> ("status"=w1472:bool)
                        }
                      }
                    }
                  }
                  frame True {
                  }
                }
                n372 = Transpose 2D Array(2D array=w1406) -> (transposed array=w1413:string[][])
                "CAP_C3" <- w1413
              }
              frame #4 {
                # "VPI Testing @ 35V"
                n373 = call "WS1050 Delta C Calculation.vi"("error in (no error)"=w1537, "DCap Target(pF)"=w1536, "Input"=w1539) -> ("error out"=w1534:errorcluster, "Total Bank Delta C(pF)"=w1527:string[], "% Bank DeltaC"=w1531:string[])  [unwired: 4 in, 2 out]
                n374 = call "WS1050 Delta C Calculation.vi"("error in (no error)"=w1537, "DCap Target(pF)"=w1536, "Input"=w1538) -> ("error out"=w1535:errorcluster, "Total Bank Delta C(pF)"=w1526:string[], "% Bank DeltaC"=w1529:string[])  [unwired: 4 in, 2 out]
                n375 = call "WS1050 Delta C Calculation.vi"("error in (no error)"=w1537, "DCap Target(pF)"=w1536, "Input"=w1530) -> ("error out"=w1533:errorcluster, "Total Bank Delta C(pF)"=w1525:string[], "% Bank DeltaC"=w1528:string[])  [unwired: 4 in, 2 out]
                n376 = Merge Errors(w1534, w1535, w1533) -> (w1532:errorcluster)
                n377 = case shown="1, Default" w1540 {
                  tunnel: w1532 -> [w1738 w1746]
                  tunnel: [w1738 w1746] -> w1499
                  tunnel: w1531 -> [w1734 w1742]
                  tunnel: w1529 -> [w1733 w1741]
                  tunnel: w1528 -> [w1732 w1740]
                  tunnel: w1527 -> [w1737 w1745]
                  tunnel: [w1737 w1745] -> w1524
                  tunnel: w1526 -> [w1736 w1744]
                  tunnel: [w1736 w1744] -> w1523
                  tunnel: w1525 -> [w1735 w1743]
                  tunnel: [w1735 w1743] -> w1522
                  frame 0 {
                    n378 = Build Array(w1734, w1733, w1732) -> (→"% Delta C_T0":string[][])
                  }
                  frame 1, Default {
                    n379 = Build Array(w1742, w1741, w1740) -> (→"% Delta C":string[][])
                  }
                }
                "Total Delta C1(pF)" <- w1524
                "Total Delta C2(pF)" <- w1523
                "Total Delta C3(pF)" <- w1522
                n380 = call "WS1050_51 VPI Header.vi"("VPI Name"="VPI Name", "VPI_Cmd"="VPI_Cmd", "Cmin/Act"=w1497, "WS1050/51"=w1508, "error in (no error)"=w1509) -> ("VPI_1"=w1507:string[], "VPI_2"=w1505:string[], "VPI Header"=w1506:string[], "VPI_3"=w1504:string[], "Cmd_3"=w1501:string[], "Cmd_1"=w1503:string[], "Cmd_2"=w1502:string[], "error out"=w1500:errorcluster)  [unwired: 3 in]
                n381 = Merge Errors(w1500, w1499) -> (w1498:errorcluster)
                n382 = case shown="False" w1496 {
                  tunnel: [w1567 w1722] -> w1552
                  tunnel: [w1566 w1722] -> w1551
                  tunnel: w1547 -> [w1565 w1720]
                  tunnel: [w1564 w1720] -> w1546
                  tunnel: [w1563 w1722] -> w1543
                  tunnel: [w1562 "" ("Data Out")] -> w1520
                  tunnel: [w1561 w1721] -> w1518
                  tunnel: w1514 -> [w1560 _]
                  tunnel: w1507 -> [w1559 _]
                  tunnel: w1505 -> [w1558 _]
                  tunnel: w1504 -> [w1557 _]
                  tunnel: w1503 -> [w1556 _]
                  tunnel: w1502 -> [w1555 _]
                  tunnel: w1501 -> [w1554 _]
                  tunnel: w1498 -> [w1553 w1721]
                  frame False {
                    n383 = case shown="False" w1560 {
                      tunnel: [w1570 w1591] -> w1561
                      tunnel: [w1568 w1609] -> w1567
                      tunnel: [w1568 w1595] -> w1566
                      tunnel: w1565 -> [w1575 w1608]
                      tunnel: [w1575 w1608] -> w1564
                      tunnel: w1556 -> [_ w1607]
                      tunnel: w1555 -> [_ w1601]
                      tunnel: w1554 -> [_ w1597]
                      tunnel: [w1568 w1606] -> w1563
                      tunnel: w1559 -> [w1573 w1604]
                      tunnel: w1558 -> [_ w1602]
                      tunnel: w1557 -> [_ w1598]
                      tunnel: ["NA" ("string") w1585] -> w1562
                      tunnel: w1553 -> [w1571 w1589]
                      frame False {
                        n384 = Array Size(array=w1573) -> (size(s)=w1572:i32)
                        n385 = for {
                          N: w1572 -> [_]
                          tunnel: [w1577] -> w1569 mode=indexing
                          tunnel: w1571 -> [w1576]
                          tunnel: [w1576] -> w1570
                          n386 = for {
                            N: 36 -> [_]
                            tunnel: [""] -> w1577 mode=indexing
                          }
                        }
                        n387 = Transpose 2D Array(2D array=w1569) -> (transposed array=w1568:string[][])
                        n388 = local write "VPI C1"(w1568) -> ()
                        n389 = local write "VPI C2"(w1568) -> ()
                        n390 = local write "VPI C3"(w1568) -> ()
                      }
                      frame True {
                        w1590 = FALSE ("Log (T)")
                        # "Set CP VPI"
                        n391 = call "WSVCAP SHL Host TL RFFE Write - Multiple DUTs - Common Data.vi"("Data Out"="074820", "error in"=w1589, "Log (T)"=w1590) -> ("error out"=w1587:errorcluster)  [unwired: 12 in]
                        n392 = call "Delay.vi"("milliseconds to wait"=u32 10, "error in (no error)"=w1587) -> ("error out"=w1583:errorcluster)  [unwired: 9 in]
                        n393 = case shown="0, Default" "CP VPI" {
                          selector: "CP VPI" -> [w1614 w1619 w1624 w1629 w1634 w1639 w1644 w1649 w1653]
                          tunnel: string[] ["07476F", "074776", "074765", "074769", "07477B", "07477C", "07477D", "074779", "07476B"] -> [w1615 w1620 w1625 w1630 w1635 w1640 w1645 w1650 w1655]
                          tunnel: [w1613 w1618 w1623 w1628 w1633 w1638 w1643 w1648 w1654] -> w1582
                          tunnel: ["35.0" ("Data Out") "27.5" ("Data Out") "30.5" ("Data Out") "44.0" ("Data Out") "50.0" ("Data Out") "55.0" ("Data Out") "42.5" ("Data Out") "32.0" ("Data Out") "40.25" ("Data Out")] -> w1585
                          tunnel: [w1611 w1616 w1621 w1626 w1631 w1636 w1641 w1646 w1651] -> w1584
                          tunnel: w1583 -> [w1611 w1616 w1621 w1626 w1631 w1636 w1641 w1646 w1651]
                          frame 0, Default {
                            n394 = Index Array(array=w1615, index=w1614) -> (element=w1613:string)
                          }
                          frame 2 {
                            n395 = Index Array(array=w1620, index=w1619) -> (element=w1618:string)
                          }
                          frame 3 {
                            n396 = Index Array(array=w1625, index=w1624) -> (element=w1623:string)
                          }
                          frame 4 {
                            n397 = Index Array(array=w1630, index=w1629) -> (element=w1628:string)
                          }
                          frame 5 {
                            n398 = Index Array(array=w1635, index=w1634) -> (element=w1633:string)
                          }
                          frame 6 {
                            n399 = Index Array(array=w1640, index=w1639) -> (element=w1638:string)
                          }
                          frame 7 {
                            n400 = Index Array(array=w1645, index=w1644) -> (element=w1643:string)
                          }
                          frame 8 {
                            n401 = Index Array(array=w1650, index=w1649) -> (element=w1648:string)
                          }
                          frame 1 {
                            n402 = Index Array(array=w1655, index=w1653) -> (element=w1654:string)
                          }
                        }
                        n403 = Array Size(array=w1604) -> (size(s)=w1610:i32)
                        n404 = call "WSVCAP SHL Host TL RFFE Write - Multiple DUTs - Common Data.vi"("Data Out"=w1582, "error in"=w1584, "Log (T)"=w1590) -> ("error out"=w1594:errorcluster)  [unwired: 12 in]
                        n405 = for {
                          N: w1610 -> [_]
                          tunnel: w1607 -> [w1714]
                          tunnel: [w1712] -> w1605 mode=indexing
                          tunnel: w1604 -> [w1711]
                          tunnel: w1594 -> [w1700]
                          tunnel: [w1702] -> w1593
                          i -> [w1710]
                          stop <- w1698 stop-if-true
                          n406 = Index Array(array=w1714, index=w1710) -> (element=w1713:string)
                          n407 = Index Array(array=w1711, index=w1710) -> (element=w1709:string)
                          n408 = local write "STATUS"(w1709) -> ()
                          n409 = call "WSVCAP SHL Host TL RFFE Write - Multiple DUTs - Common Data.vi"("Data Out"=w1713, "error in"=w1700, "Log (T)"=FALSE) -> ("error out"=w1708:errorcluster)  [unwired: 12 in]
                          n410 = call "Delay.vi"("milliseconds to wait"=u32 10, "error in (no error)"=w1708) -> ("error out"=w1704:errorcluster)  [unwired: 9 in]
                          n411 = call "WS1050 AD7747 READ 36 DUT.vi"("error in"=w1704, "Log (T)"=FALSE, "DUT Mask Mode (All)"=WSVCAP_SHL_I2C_DUT_Mask_Mode_Enum."C1") -> ("error out"=w1706:errorcluster, "AD7747 Values"=w1705:string[][])  [unwired: 7 in]
                          n412 = for {
                            tunnel: [w1717] -> w1712 mode=indexing
                            tunnel: w1706 -> [w1716]
                            tunnel: [w1716] -> w1702
                            tunnel: w1705 -> [w1715] mode=indexing
                            n413 = Index Array(array=w1715, index=1) -> (element=w1717:string)
                          }
                          n414 = Unbundle By Name(w1702) -> ("status"=w1698:bool)
                        }
                        n415 = Transpose 2D Array(2D array=w1605) -> (transposed array=w1609:string[][])
                        "VPI C1" <- w1609
                        n416 = Array Size(array=w1602) -> (size(s)=w1603:i32)
                        n417 = for {
                          N: w1603 -> [_]
                          tunnel: w1601 -> [w1693]
                          tunnel: [w1691] -> w1600 mode=indexing
                          tunnel: w1602 -> [w1690]
                          tunnel: w1593 -> [w1679]
                          tunnel: [w1681] -> w1592
                          i -> [w1689]
                          stop <- w1677 stop-if-true
                          n418 = Index Array(array=w1693, index=w1689) -> (element=w1692:string)
                          n419 = Index Array(array=w1690, index=w1689) -> (element=w1688:string)
                          n420 = call "WSVCAP SHL Host TL RFFE Write - Multiple DUTs - Common Data.vi"("Data Out"=w1692, "error in"=w1679, "Log (T)"=FALSE) -> ("error out"=w1687:errorcluster)  [unwired: 12 in]
                          n421 = local write "STATUS"(w1688) -> ()
                          n422 = call "Delay.vi"("milliseconds to wait"=u32 10, "error in (no error)"=w1687) -> ("error out"=w1683:errorcluster)  [unwired: 9 in]
                          n423 = call "WS1050 AD7747 READ 36 DUT.vi"("error in"=w1683, "Log (T)"=FALSE, "DUT Mask Mode (All)"=WSVCAP_SHL_I2C_DUT_Mask_Mode_Enum."C2") -> ("error out"=w1685:errorcluster, "AD7747 Values"=w1684:string[][])  [unwired: 7 in]
                          n424 = for {
                            tunnel: [w1696] -> w1691 mode=indexing
                            tunnel: w1685 -> [w1695]
                            tunnel: [w1695] -> w1681
                            tunnel: w1684 -> [w1694] mode=indexing
                            n425 = Index Array(array=w1694, index=3) -> (element=w1696:string)
                          }
                          n426 = Unbundle By Name(w1681) -> ("status"=w1677:bool)
                        }
                        n427 = Transpose 2D Array(2D array=w1600) -> (transposed array=w1606:string[][])
                        "VPI C2" <- w1606
                        n428 = Array Size(array=w1598) -> (size(s)=w1599:i32)
                        n429 = for {
                          N: w1599 -> [_]
                          tunnel: w1597 -> [w1672]
                          tunnel: [w1670] -> w1596 mode=indexing
                          tunnel: w1598 -> [w1669]
                          tunnel: w1592 -> [w1658]
                          tunnel: [w1660] -> w1591
                          i -> [w1668]
                          stop <- w1656 stop-if-true
                          n430 = Index Array(array=w1672, index=w1668) -> (element=w1671:string)
                          n431 = Index Array(array=w1669, index=w1668) -> (element=w1667:string)
                          n432 = call "WSVCAP SHL Host TL RFFE Write - Multiple DUTs - Common Data.vi"("Data Out"=w1671, "error in"=w1658, "Log (T)"=FALSE) -> ("error out"=w1666:errorcluster)  [unwired: 12 in]
                          n433 = local write "STATUS"(w1667) -> ()
                          n434 = call "Delay.vi"("milliseconds to wait"=u32 10, "error in (no error)"=w1666) -> ("error out"=w1662:errorcluster)  [unwired: 9 in]
                          n435 = call "WS1050 AD7747 READ 36 DUT.vi"("error in"=w1662, "Log (T)"=FALSE, "DUT Mask Mode (All)"=WSVCAP_SHL_I2C_DUT_Mask_Mode_Enum."C3") -> ("error out"=w1664:errorcluster, "AD7747 Values"=w1663:string[][])  [unwired: 7 in]
                          n436 = for {
                            tunnel: [w1675] -> w1670 mode=indexing
                            tunnel: w1664 -> [w1674]
                            tunnel: [w1674] -> w1660
                            tunnel: w1663 -> [w1673] mode=indexing
                            n437 = Index Array(array=w1673, index=5) -> (element=w1675:string)
                          }
                          n438 = Unbundle By Name(w1660) -> ("status"=w1656:bool)
                        }
                        n439 = Transpose 2D Array(2D array=w1596) -> (transposed array=w1595:string[][])
                        "VPI C3" <- w1595
                      }
                    }
                  }
                  frame True {
                    w1722 = string[][] []
                  }
                }
                n440 = Insert Into Array(array=w1542, new element=w1506) -> (w1541:string[])  [unwired: 1 in]
                n441 = case shown="True" w1519 {
                  tunnel: w1518 -> [w1724 w1729]
                  tunnel: [w1725 w1728] -> w1517
                  frame False {
                    n442 = call "WSVCAP SHL Host TL RFFE Write - Multiple DUTs - Common Data.vi"("Data Out"="074820", "error in"=w1724, "Log (T)"=FALSE) -> ("error out"=w1725:errorcluster)  [unwired: 12 in]
                  }
                  frame True {
                    n443 = call "WSVCAP SHL Host TL RFFE Write - Multiple DUTs - Common Data.vi"("Data Out"="074800", "error in"=w1729, "Log (T)"=FALSE) -> ("error out"=w1728:errorcluster)  [unwired: 12 in]
                  }
                }
                n444 = call "Delay.vi"("milliseconds to wait"=u32 10, "error in (no error)"=w1517) -> ("error out"=w1516:errorcluster)  [unwired: 9 in]
              }
              frame #5 {
                # "VSA Testing"
                n445 = case shown="True" w1748 {
                  tunnel: w1788 -> [w1798 w1868]
                  tunnel: w1779 -> [w1797 w1867]
                  tunnel: [w1796 w1867] -> w1778
                  tunnel: [w1795 string[][] []] -> w1768
                  tunnel: [w1794 w1869] -> w1767
                  tunnel: [w1793 w1869] -> w1764
                  tunnel: [w1792 w1868] -> w1762
                  tunnel: [w1791 w1869] -> w1761
                  tunnel: w1749 -> [w1790 _]
                  frame False {
                    n446 = case shown="True" w1790 {
                      tunnel: w1798 -> [w1800 w1814]
                      tunnel: [w1799 w1813] -> w1792
                      tunnel: [w1804 w1820] -> w1796
                      tunnel: w1797 -> [w1804 w1819]
                      tunnel: [w1801 w1817] -> w1794
                      tunnel: [w1801 w1816] -> w1793
                      tunnel: [w1801 w1815] -> w1791
                      tunnel: [w1802 w1818] -> w1795
                      frame False {
                        n447 = for {
                          tunnel: dbl[] [0.0, 0.0, 0.0] -> [w1809] mode=indexing
                          tunnel: [w1808] -> w1802 mode=indexing
                          tunnel: [w1805] -> w1801 mode=indexing
                          tunnel: w1800 -> [w1806]
                          tunnel: [w1806] -> w1799
                          n448 = Number To Fractional String(number=w1809) -> (F-format string=w1810:string)  [unwired: 3 in]
                          n449 = for {
                            N: 36 -> [_]
                            tunnel: w1810 -> [w1812]
                            tunnel: [w1812] -> w1808 mode=indexing
                            tunnel: [""] -> w1805 mode=indexing
                          }
                        }
                      }
                      frame True {
                        n450 = for {
                          tunnel: "VSA Voltage(V)" -> [w1844] mode=indexing
                          tunnel: [w1848] -> w1820
                          tunnel: w1819 -> [w1846]
                          tunnel: [w1845] -> w1817 mode=indexing
                          tunnel: [w1832] -> w1816 mode=indexing
                          tunnel: [w1841] -> w1818 mode=indexing
                          tunnel: [w1826] -> w1815 mode=indexing
                          tunnel: w1814 -> [w1825]
                          tunnel: [w1824] -> w1813
                          w1823 = FALSE ("Log (T)")
                          w1840 = u16 0 items=["Voltage", "Current"] ("Source Mode  (0: Voltage)")
                          n451 = call "Ke2400 Configure Output.vi"("Source Mode  (0: Voltage)"=w1840, "error in (no error)"=w1825, "Compliance  Level (0.1)"=0.1, "Output Level (0)"=w1844, "VISA resource name"=w1846) -> ("error out"=w1852:errorcluster, "VISA resource name out"=w1850:refnum<visa-resource-name>)  [unwired: 5 in]
                          n452 = Number To Fractional String(number=w1844) -> (F-format string=w1843:string)  [unwired: 3 in]
                          n453 = call "Ke2400 Enable.vi"("error in (no error)"=w1852, "ON/OFF"=TRUE ("Enable Output (T: Enable)"), "VISA resource name"=w1850) -> ("error out"=w1853:errorcluster, "VISA resource name out"=w1848:refnum<visa-resource-name>)  [unwired: 7 in]
                          n454 = call "Delay.vi"("milliseconds to wait"=u32 10, "error in (no error)"=w1853) -> ("error out"=w1839:errorcluster)  [unwired: 9 in]
                          n455 = call "WS1050 AD7747 READ 36 DUT.vi"("error in"=w1839, "Log (T)"=w1823, "DUT Mask Mode (All)"=WSVCAP_SHL_I2C_DUT_Mask_Mode_Enum."C1") -> ("error out"=w1836:errorcluster, "AD7747 Values"=w1838:string[][])  [unwired: 7 in]
                          n456 = for {
                            tunnel: w1838 -> [w1864] mode=indexing
                            tunnel: [w1865] -> w1845 mode=indexing
                            tunnel: w1836 -> [w1863]
                            tunnel: [w1863] -> w1835
                            n457 = Index Array(array=w1864, index=1) -> (element=w1865:string)
                          }
                          n458 = for {
                            N: 36 -> [_]
                            tunnel: w1843 -> [w1862]
                            tunnel: [w1862] -> w1841 mode=indexing
                          }
                          n459 = call "WS1050 AD7747 READ 36 DUT.vi"("error in"=w1835, "Log (T)"=w1823, "DUT Mask Mode (All)"=WSVCAP_SHL_I2C_DUT_Mask_Mode_Enum."C2") -> ("error out"=w1833:errorcluster, "AD7747 Values"=w1831:string[][])  [unwired: 7 in]
                          n460 = for {
                            tunnel: w1831 -> [w1859] mode=indexing
                            tunnel: [w1860] -> w1832 mode=indexing
                            tunnel: w1833 -> [w1858]
                            tunnel: [w1858] -> w1830
                            n461 = Index Array(array=w1859, index=3) -> (element=w1860:string)
                          }
                          n462 = call "WS1050 AD7747 READ 36 DUT.vi"("error in"=w1830, "Log (T)"=w1823, "DUT Mask Mode (All)"=WSVCAP_SHL_I2C_DUT_Mask_Mode_Enum."C3") -> ("error out"=w1828:errorcluster, "AD7747 Values"=w1827:string[][])  [unwired: 7 in]
                          n463 = local write "STATUS"("VSA Testing...." ("STATUS")) -> ()
                          n464 = for {
                            tunnel: w1827 -> [w1855] mode=indexing
                            tunnel: [w1856] -> w1826 mode=indexing
                            tunnel: w1828 -> [w1854]
                            tunnel: [w1854] -> w1824
                            n465 = Index Array(array=w1855, index=5) -> (element=w1856:string)
                          }
                        }
                      }
                    }
                  }
                  frame True {
                    w1869 = string[][] []
                  }
                }
                n466 = Transpose 2D Array(2D array=w1768) -> (transposed array=w1766:string[][])
                n467 = Transpose 2D Array(2D array=w1767) -> (transposed array=w1765:string[][])
                n468 = Transpose 2D Array(2D array=w1764) -> (transposed array=w1763:string[][])
                n469 = Transpose 2D Array(2D array=w1761) -> (transposed array=w1760:string[][])
                n470 = call "WS1050_VSA_Convert_Data.vi"("VSA_C3"=w1760, "error in (no error)"=w1762, "VSA_C2"=w1763, "VSA_C1"=w1765, "Voltage"=w1766) -> ("error out"=w1759:errorcluster, "VSA_V3"=w1756:string[][], "VSA_V2"=w1757:string[][], "VSA_V1"=w1758:string[][])  [unwired: 3 in]
                "VSA_V1" <- w1758
                "VSA_V2" <- w1757
                "VSA_V3" <- w1756
                n471 = case shown="True" w1749 {
                  tunnel: w1778 -> [w1872 w1878]
                  tunnel: [w1872 w1877] -> w1777
                  tunnel: w1759 -> [w1871 w1876]
                  tunnel: [w1871 w1873] -> w1776
                  frame False {
                  }
                  frame True {
                    w1874 = u16 0 items=["Voltage", "Current"] ("Source Mode  (0: Voltage)")
                    n472 = call "Ke2400 Configure Output.vi"("Source Mode  (0: Voltage)"=w1874, "error in (no error)"=w1876, "Output Level (0)"=0.0, "VISA resource name"=w1878) -> ("error out"=w1873:errorcluster, "VISA resource name out"=w1877:refnum<visa-resource-name>)  [unwired: 6 in]
                  }
                }
                n473 = call "Delay.vi"("milliseconds to wait"=u32 50, "error in (no error)"=w1776) -> ("error out"=w1775:errorcluster)  [unwired: 9 in]
              }
              frame #6 {
                # "Handshake Check and EFuse Readback"
                n474 = Or(x=w1888, y=w1898) -> (x .or. y?=w1897:bool)
                n475 = Add(x=w1910, y=w1909) -> (x+y=w1896:u64)
                n476 = case shown="True" w1897 {
                  tunnel: w1923 -> [w1936 _]
                  tunnel: w1922 -> [w1935 w1941]
                  tunnel: [w1934 w1941] -> w1921
                  tunnel: w1920 -> [w1933 _]
                  tunnel: w1919 -> [w1932 _]
                  tunnel: w1918 -> [w1931 _]
                  tunnel: [w1927 w1940] -> w1917
                  tunnel: [w1926 w1940] -> w1912
                  tunnel: w1896 -> [w1925 _]
                  tunnel: w1903 -> [w1924 _]
                  frame False {
                    n477 = call "WS1050_36DUT_Handshake Check R1_Record All Regs Ver1.0.vi"("file path (use dialog)"=w1936, "Reg1_Bit Cntrl"="Reg1_Bit Cntrl", "File Name"=w1924, "SN"=w1931, "Loop"=w1925, "error"=w1935, "Lot #"=w1933, "Wafer #"=w1932) -> ("Pass/Fail"=→"EFuse Readback Status":bool[], "EFuse Read back"=w1926:string[], "Status"=w1927:string[], "error out"=w1934:errorcluster)  [unwired: 6 in, 2 out]
                    n478 = case shown="1, Default" w1925 {
                      tunnel: w1926 -> [w1937 w1938]
                      frame 0 {
                        "EFuse RB T0" <- w1937
                      }
                      frame 1, Default {
                        "Current EFuse Read back" <- w1938
                      }
                    }
                    n479 = local write "STATUS"("Hand Shake & EFuse Readback...." ("STATUS")) -> ()
                  }
                  frame True {
                    n480 = for {
                      N: 36 -> [_]
                      tunnel: [""] -> w1940 mode=indexing
                    }
                  }
                }
                n481 = Add(x=w1896, y=w1893) -> (x+y=w1894:u64)
                "TTCompleted" <- w1894
                n482 = Number To Engineering String(4:w1894) -> (0:w1908:string)  [unwired: 3 in]
                n483 = Build Array(w1907, w1905, w1904) -> (w1906:string[])
              }
              frame #7 {
                # "Save Data"
                n484 = Increment(x=w1959) -> (x+1=w1958:i32)
                n485 = Multiply(x=w1958, y=36) -> (x*y=w1953:i32)
                n486 = Path To String(path=w1947) -> (string=w1962:string)
                n487 = Bundle("Test Program"=w1992, "Comment"=w1991, "Data Out"=w1969, "Data Out"=w1968, "Data Out"=w1967, w1966, "Data Out"=w1965, "Data Out"=w1964, "Data Out"=w1963, "Freq(Hz)"=w1951, "Board#"=w1946) -> (w1950:T8)  [unwired: 1 in]
                n488 = case shown="False" w1949 {
                  tunnel: w1997 -> [w2024 w2026]
                  tunnel: [w2023 w2026] -> w1996
                  tunnel: w1995 -> [w2022 _]
                  tunnel: w1994 -> [w2021 _]
                  tunnel: w1993 -> [w2020 _]
                  tunnel: w1990 -> [w2019 _]
                  tunnel: w1988 -> [w2018 _]
                  tunnel: w1987 -> [w2017 _]
                  tunnel: w1986 -> [w2016 _]
                  tunnel: w1985 -> [w2015 _]
                  tunnel: w1984 -> [w2014 _]
                  tunnel: w1981 -> [w2013 _]
                  tunnel: w1980 -> [w2012 _]
                  tunnel: w1979 -> [w2011 _]
                  tunnel: w1944 -> [w2010 _]
                  tunnel: w1977 -> [w2009 _]
                  tunnel: w1976 -> [w2008 _]
                  tunnel: w1975 -> [w2007 _]
                  tunnel: w1974 -> [w2006 _]
                  tunnel: w1973 -> [w2005 _]
                  tunnel: w1972 -> [w2004 _]
                  tunnel: w1971 -> [w2003 _]
                  tunnel: w1970 -> [w2002 _]
                  tunnel: w1947 -> [w2001 _]
                  tunnel: w1956 -> [w2000 _]
                  tunnel: w1950 -> [w1999 _]
                  tunnel: ["Save Data...." ("STATUS") "Stop test..." ("STATUS")] -> w1948
                  frame False {
                    n489 = call "WS1050_36 DUT SData Ver1.0.vi"("TMN DC\\CAP Data Log File Path"=w2001, "Lot#"=w2021, "Total Delta C1(pF)"=w2004, "VSA_V1"=w2012, "Wafer#"=w2019, "File Name"=w2000, "Total Delta C2(pF)"=w2003, "error in"=w2024, "TP/Comment"=w1999, "EFuse"=w2015, "Data Output C3"=w2006, "Temperature"=w2010, "VSA_V2"=w2013, "VPI C3"=w2008, "Data Output C1"=w2018, "VPI C2"=w2007, "SN"=w2022, "R/W Status"=w2020, "Cap Header"=w2009, "HD/Cycles Completed"=w2014, "Data Output C2"=w2005, "VSA_V3"=w2011, "Current"=w2017, "VPI C1"=w2016, "Total Delta C3(pF)"=w2002) -> ("error out"=w2023:errorcluster)  [unwired: 2 in]
                  }
                  frame True {
                  }
                }
                n490 = case shown="True" "Debug" {
                  tunnel: w1953 -> [w2027 w2030]
                  tunnel: [w2027 w2028] -> w1952
                  frame False {
                  }
                  frame True {
                    n491 = Multiply(x=w2030, y="No of Rows\nFrom Spread Sheet") -> (x*y=w2028:i32)
                  }
                }
                n492 = local write "STATUS"(w1948) -> ()
                n493 = Concatenate Strings(w1962, "\\" ("string"), w1956, "_Multi Socket Data.csv" ("string")) -> (w1961:string)
              }
              frame #8 {
                n494 = case shown="True" "Plot Delta Cmin" {
                  tunnel: w2045 -> [w2058 w2073]
                  tunnel: [w2058 w2069] -> w2044
                  tunnel: w2043 -> [_ w2065]
                  tunnel: w2041 -> [_ w2063]
                  frame False {
                  }
                  frame True {
                    n495 = String To Path(string=w2065) -> (path=w2064:path)
                    n496 = call "Delay.vi"("milliseconds to wait"=u32 50, "error in (no error)"=w2073) -> ("error out"=w2072:errorcluster)  [unwired: 9 in]
                    n497 = call "36DUT Plot From Spread Sheet.vi"("Plot"="Plot", "No of Rows"=w2063, "error in (no error)"=w2072, "Bank"="Bank C1", "file path (dialog if empty)"=w2064) -> ("error out"=w2067:errorcluster, "Delta C_Min Plot"=→"Min Plot_1":dbl[][])  [unwired: 5 in]
                    n498 = call "36DUT Plot From Spread Sheet.vi"("Plot"="Plot", "No of Rows"=w2063, "error in (no error)"=w2067, "Bank"="Bank C2", "file path (dialog if empty)"=w2064) -> ("error out"=w2068:errorcluster, "Delta C_Min Plot"=→"Min Plot_2":dbl[][])  [unwired: 5 in]
                    n499 = call "36DUT Plot From Spread Sheet.vi"("Plot"="Plot", "No of Rows"=w2063, "error in (no error)"=w2068, "Bank"="Bank C3", "file path (dialog if empty)"=w2064) -> ("error out"=w2069:errorcluster, "Delta C_Min Plot"=→"Min Plot_3":dbl[][])  [unwired: 5 in]
                  }
                }
                n500 = Get Date/Time In Seconds() -> (seconds since 1Jan1904=w2051:timestamp)
                n501 = Get Date/Time String(seconds (now)=w2051, want seconds? (F)=TRUE) -> (date string=→"date string":string, time string=→"Previous Time":string)  [unwired: 1 in]
                n502 = Greater Or Equal?(x=w2039, y="Set HD/Cycle \nto Complete") -> (x >= y?=w2055:bool)
                n503 = Greater Or Equal?(x=w2048, y="TTF Completed") -> (x >= y?=w2047:bool)
                "No of HD/Cycle\nCompleted" <- w2039
              }
              frame #9 {
                n504 = case shown="True" w2079 {
                  tunnel: w2095 -> [w2104 w2127]
                  tunnel: w2094 -> [_ w2115]
                  tunnel: w2075 -> [_ w2128]
                  tunnel: [w2104 w2125] -> w2093
                  tunnel: w2092 -> [_ w2124]
                  tunnel: w2091 -> [_ w2123]
                  tunnel: w2090 -> [_ w2122]
                  tunnel: w2089 -> [_ w2121]
                  tunnel: w2088 -> [_ w2120]
                  tunnel: w2086 -> [_ w2119]
                  tunnel: w2087 -> [_ w2118]
                  tunnel: w2076 -> [_ w2117]
                  tunnel: w2085 -> [w2103 w2112]
                  tunnel: [w2103 w2111] -> w2084
                  tunnel: w2083 -> [w2102 w2110]
                  tunnel: [w2102 w2109] -> w2082
                  tunnel: w2081 -> [w2101 w2108]
                  tunnel: [w2101 w2107] -> w2080
                  tunnel: w2078 -> [_ w2106]
                  tunnel: w2077 -> [_ w2105]
                  frame False {
                  }
                  frame True {
                    n505 = call "Read Point CP CV Sweep.vi"("error in"=w2127, "Numeric"=w2115, "Set Point for\nCV CV Sweep"=w2128) -> ("error Out"=w2126:errorcluster, "Last Number"=w2113:u64, "Ind"=w2116:bool)  [unwired: 4 in, 2 out]
                    n506 = Number To Exponential String(number=w2113) -> (E-format string=w2114:string)  [unwired: 3 in]
                    n507 = case shown="True" w2116 {
                      tunnel: w2126 -> [w2132 w2156]
                      tunnel: [w2132 w2155] -> w2125
                      tunnel: w2124 -> [_ w2154]
                      tunnel: w2123 -> [_ w2153]
                      tunnel: w2122 -> [_ w2152]
                      tunnel: w2121 -> [_ w2151]
                      tunnel: w2120 -> [_ w2150]
                      tunnel: w2119 -> [_ w2149]
                      tunnel: w2118 -> [_ w2148]
                      tunnel: w2117 -> [_ w2147]
                      tunnel: w2114 -> [_ w2146]
                      tunnel: w2112 -> [w2131 w2141]
                      tunnel: [w2131 w2140] -> w2111
                      tunnel: w2110 -> [w2130 w2139]
                      tunnel: [w2130 w2138] -> w2109
                      tunnel: w2108 -> [w2129 w2137]
                      tunnel: [w2129 w2136] -> w2107
                      tunnel: w2106 -> [_ w2134]
                      tunnel: w2105 -> [_ w2133]
                      frame False {
                      }
                      frame True {
                        n508 = call "WS1050 36 DUT CP CV Sweep SubVI.vi"("TMN DC\\CAP Data Log File Path"=w2154, "Test Program"=w2152, "Lot#"=w2151, "Wafer#"=w2150, "Board#"=w2148, "Temp"=w2134, "error in (no error)"=w2156, "File Name"=w2149, "Comment"=w2133, "Ke2400"=w2141, "PS1 Source"=w2137, "Serial Number"=w2153, "CP Set to Run"=w2147, "HD/Cycles Completed"=w2146, "Ke2000"=w2139) -> ("Plot_1"=→"CP CV Sweep C1":dbl[][], "Plot_2"=→"CP CV Sweep C2":dbl[][], "Ke2400 Out"=w2140:refnum<visa-resource-name>, "Plot_3"=→"CP CV Sweep C3":dbl[][], "CP Voltage"=→"LP CP Voltage":string, "PS1 Out"=w2136:refnum<visa-resource-name>, "Ke2000 Out"=w2138:refnum<visa-resource-name>, "error out"=w2155:errorcluster)  [unwired: 2 in, 3 out]
                        n509 = local write "STATUS"("CP CV Sweep..." ("STATUS")) -> ()
                      }
                    }
                  }
                }
              }
            }
            n510 = Concatenate Strings("File Name", "_CP CV Sweep" ("string")) -> (w503:string)
            n511 = Increment(x=w680) -> (x+1=→"Loop \ncompleted":i32)
            n512 = call "Delay.vi"("milliseconds to wait"=u32 10, "error in (no error)"=w570) -> ("error out"=w571:errorcluster)  [unwired: 9 in]
            n513 = Compound Arithmetic op=OR(w748, w650, w676) -> (w689:bool)
          }
          "Total Time" <- w477
          n514 = Increment(x=w475) -> (x+1=→"Run Loops":i32)
          n515 = local write "No of HD/Cycle\nCompleted"(u64 0 ("No of HD/Cycle\nCompleted")) -> ()
          n516 = Unbundle By Name(w467) -> ("status"=w481:bool)
          n517 = Compound Arithmetic op=OR(w481, w473, w472) -> (w451:bool)
        }
        n518 = flat-sequence {
          tunnel: w306 -> [w374]
          tunnel: [w374] -> w305
          tunnel: w304 -> [w373]
          tunnel: [w373] -> w303
          frame #0 {
            n519 = local write "STATUS"("Completed!" ("STATUS")) -> ()
            n520 = One Button Dialog(message="Done!") -> ()  [unwired: 1 in, 1 out]
          }
        }
        n521 = for {
          tunnel: w332 -> [w2167]
          tunnel: w313 -> [w2166]
          tunnel: w361 -> [w2164] mode=indexing
          tunnel: [w2159] -> w331
          tunnel: [w2163] -> w360
          n522 = call "E3631A_Voltage Controller updated.vi"("VISA resource name"=w2166, "I_VDD(A)"=0.5, "Channel Controller"=w2164, "Voltage 1"=0.0, "Voltage 2"=3.3, "error in (no error)"=w2167, "I_3.3V (A)"=0.5) -> ("VISA resource name out"=w2163:refnum<visa-resource-name>, "error out"=w2160:errorcluster)  [unwired: 7 in]
          n523 = call "Delay.vi"("milliseconds to wait"=u32 100, "error in (no error)"=w2160) -> ("error out"=w2159:errorcluster)  [unwired: 9 in]
        }
        n524 = VISA Write(VISA resource name=w351, write buffer="SOUR:FUNC VOLT;VOLT:MODE FIX;RANG 100;LEV 0.0;:SENS:FUNC \"CURR\";CURR:PROT 60E-3;RANG 100E-3;:OUTP ON", error in (no error)=w332) -> (VISA resource name out=w349:refnum<visa-resource-name>, error out=w304:errorcluster)  [unwired: 1 out]
        n525 = Merge Errors(w331, w303) -> (w350:errorcluster)
      }
      frame True {
        w2179 = FALSE ("stop During HD/Cycles")
      }
    }
    n526 = Unbundle By Name(w75) -> ("status"=w74:bool)
    n527 = Compound Arithmetic op=OR(w73, w74, w95) -> (w103:bool)
    n528 = Wait Until Next ms Multiple(millisecond multiple=u32 100) -> ()  [unwired: 1 out]
    "STATUS" <- "Idle...." ("STATUS")
  }
  "Ke2000 Out" <- w11
  n529 = local write "stop During HD/Cycles"(w17) -> ()
  n530 = local write "stop"(w17) -> ()
  n531 = case shown="True" w26 {
    tunnel: [w2184 w2187] -> w9
    tunnel: w5 -> [w2184 w2186]
    frame False {
    }
    frame True {
      n532 = local write "Online"(FALSE ("Online")) -> ()
      n533 = call "WSVCAP SHL Host TL Close.vi"("error in"=w2186) -> ("error out"=w2187:errorcluster)  [unwired: 14 in]
    }
  }
  "error out" <- w9
  n534 = VISA Write(VISA resource name=w21, write buffer="SOUR:FUNC VOLT;VOLT:MODE FIX;RANG 100;LEV 0.0;:SENS:FUNC \"CURR\";CURR:PROT 60E-3;RANG 100E-3;:OUTP OFF", error in (no error)=w5) -> (VISA resource name out=→"VISA out":refnum<visa-resource-name>, error out=w8:errorcluster)  [unwired: 1 out]
  n535 = VISA Write(VISA resource name=w6, write buffer=":INST:NSEL 1; :VOLT 0.000000;:OUTP 1;", error in (no error)=w5) -> (VISA resource name out=→"PS1 Out":refnum<visa-resource-name>, error out=w4:errorcluster)  [unwired: 1 out]
  n536 = Merge Errors(w4, w9, w8) -> (→"error out 2":errorcluster)
